vi "(SubVI)DW7914.vi"() -> ()   [LabVIEW 2020]
uses:
  Controls/(Ctrl)DW7914_Trig Wave Ctrl.ctl
  DW7912/Controls/(Ctrl)DW7912_Wave Seq.ctl
  System Command/Controls/(Ctrl)System Command_Trig GPIO Control.ctl
  <vilib>/Utility/miscctls.llb/LVPointTypeDef.ctl
  Control Data/Controls/(Ctrl)Control Data_Save or Load Control Data_Function.ctl
  Libraries/Haptic IC Class/Haptic IC/Haptic IC.lvclass/Haptic IC.ctl
  I2C/Controls/(Ctrl)I2C_8Bit_Read Array.ctl
  Waveform Editor/Controls/(Ctrl)Waveform Editor_Update Sampling Rate Value.ctl
  a7fdcbe2-e318-4fc3-ac41-e38a3fe8abb3.vi
  26a1efa9-de36-48db-9673-265351e4b95c.vi
  Libraries/Haptic IC Class/Haptic IC/Accessors/Write freq ref.vi
  Libraries/Haptic IC Class/Haptic IC/Accessors/Write voltage range ref.vi
  Libraries/Haptic IC Class/Haptic IC/Accessors/Write mode ref.vi
  Variables/(Var)System Variables.vi
  I2C/Instance VIs/(SubVI)I2C_8Bit-8Bit_Read_Single.vi
  I2C/Instance VIs/(SubVI)I2C_8Bit-8Bit_Read_Sequential.vi
  I2C/Instance VIs/(SubVI)I2C_8Bit-8Bit_Write_Single.vi
  I2C/Instance VIs/(SubVI)I2C_8Bit-8Bit_Read_Array.vi
  I2C/Instance VIs/(SubVI)I2C_8Bit-8Bit_Write_Sequential.vi
  <vilib>/Comparison/Equal/Equal Functor/Equal Functor.lvclass
  Libraries/Haptic IC Class/Haptic IC/Haptic IC.lvclass
panel:
  in  "Stop":bool
  in  "Read All":bool
  in  "Mode Tab":T1(tab)
  in  "Mem_Brake_VD":u8(ring) caption="Brake1 M VD" items=["1.0", "0.5", "0.25", "0.25"]
  in  "Mem_Brake_Cycle 1":u8(ring) caption="Brake1 M Cycle" items=["1", "2", "3", "4", "5", "6", "7", "8"]
  in  "Mem_Brake_Cycle 0":u8(ring) caption="Brake0 M Cycle" items=["1", "2", "3", "4"]
  in  "Mem_Brake_Wave 1":u8(ring) caption="Brake1 M Wave" items=["Empty", "1", "2", "3", "4", "5", "6", "7", "8", "9", "10", "11", "12", "13", "14", "15", "16", "17", "18", "19", "20", "21", "22", "23", "24", "25", "26", "27", "28", "29", "30", "31", "32", "33", "34", "35", "36", "37", "38", "39", "40", "41", "42", "43", "44", "45", "46", "47", "48", "49", "50", "51", "52", "53", "54", "55", "56", "57", "58", "59", "60", "61", "62", "63", "64", "65", "66", "67", "68", "69", "70", "71", "72", "73", "74", "75", "76", "77", "78", "79", "80", "81", "82", "83", "84", "85", "86", "87", "88", "89", "90", "91", "92", "93", "94", "95", "96", "97", "98", "99", "100", "101", "102", "103", "104", "105", "106", "107", "108", "109", "110", "111", "112", "113", "114", "115", "116", "117", "118", "119", "120", "121", "122", "123", "124", "125", "126", "127"]
  in  "Mem_Brake_Wave 0":u8(ring) caption="Brake0 M Wave" items=["Empty", "1", "2", "3", "4", "5", "6", "7", "8", "9", "10", "11", "12", "13", "14", "15", "16", "17", "18", "19", "20", "21", "22", "23", "24", "25", "26", "27", "28", "29", "30", "31", "32", "33", "34", "35", "36", "37", "38", "39", "40", "41", "42", "43", "44", "45", "46", "47", "48", "49", "50", "51", "52", "53", "54", "55", "56", "57", "58", "59", "60", "61", "62", "63", "64", "65", "66", "67", "68", "69", "70", "71", "72", "73", "74", "75", "76", "77", "78", "79", "80", "81", "82", "83", "84", "85", "86", "87", "88", "89", "90", "91", "92", "93", "94", "95", "96", "97", "98", "99", "100", "101", "102", "103", "104", "105", "106", "107", "108", "109", "110", "111", "112", "113", "114", "115", "116", "117", "118", "119", "120", "121", "122", "123", "124", "125", "126", "127"]
  in  "Mem Set_Wave Seq Loop":T2 {"Loop 7" items=["X1", "X2", "X3", "X4", "X5", "X6", "X7", "X8", "X9", "X10", "X11", "X12", "X13", "X14", "X15", "Infinite"]; "Loop 6" items=["X1", "X2", "X3", "X4", "X5", "X6", "X7", "X8", "X9", "X10", "X11", "X12", "X13", "X14", "X15", "Infinite"]; "Loop 5" items=["X1", "X2", "X3", "X4", "X5", "X6", "X7", "X8", "X9", "X10", "X11", "X12", "X13", "X14", "X15", "Infinite"]; "Loop 4" items=["X1", "X2", "X3", "X4", "X5", "X6", "X7", "X8", "X9", "X10", "X11", "X12", "X13", "X14", "X15", "Infinite"]; "Loop 3" items=["X1", "X2", "X3", "X4", "X5", "X6", "X7", "X8", "X9", "X10", "X11", "X12", "X13", "X14", "X15", "Infinite"]; "Loop 2" items=["X1", "X2", "X3", "X4", "X5", "X6", "X7", "X8", "X9", "X10", "X11", "X12", "X13", "X14", "X15", "Infinite"]; "Loop 1" items=["X1", "X2", "X3", "X4", "X5", "X6", "X7", "X8", "X9", "X10", "X11", "X12", "X13", "X14", "X15", "Infinite"]; "Loop 0" items=["X1", "X2", "X3", "X4", "X5", "X6", "X7", "X8", "X9", "X10", "X11", "X12", "X13", "X14", "X15", "Infinite"]}
  in  "Mem_Stop":bool
  in  "Mem_Start":bool
  in  "Mem_Wave Seq":T4 caption="WAVE SEQUENCE" {"Wave Seq. 7"."Seq/Delay" items=["Empty", "1", "2", "3", "4", "5", "6", "7", "8", "9", "10", "11", "12", "13", "14", "15", "16", "17", "18", "19", "20", "21", "22", "23", "24", "25", "26", "27", "28", "29", "30", "31", "32", "33", "34", "35", "36", "37", "38", "39", "40", "41", "42", "43", "44", "45", "46", "47", "48", "49", "50", "51", "52", "53", "54", "55", "56", "57", "58", "59", "60", "61", "62", "63", "64", "65", "66", "67", "68", "69", "70", "71", "72", "73", "74", "75", "76", "77", "78", "79", "80", "81", "82", "83", "84", "85", "86", "87", "88", "89", "90", "91", "92", "93", "94", "95", "96", "97", "98", "99", "100", "101", "102", "103", "104", "105", "106", "107", "108", "109", "110", "111", "112", "113", "114", "115", "116", "117", "118", "119", "120", "121", "122", "123", "124", "125", "126", "127"]; "Wave Seq. 7"."Mode" items=["Wave Seq. 7", "Delay"]; "Wave Seq. 6"."Seq/Delay" items=["Empty", "1", "2", "3", "4", "5", "6", "7", "8", "9", "10", "11", "12", "13", "14", "15", "16", "17", "18", "19", "20", "21", "22", "23", "24", "25", "26", "27", "28", "29", "30", "31", "32", "33", "34", "35", "36", "37", "38", "39", "40", "41", "42", "43", "44", "45", "46", "47", "48", "49", "50", "51", "52", "53", "54", "55", "56", "57", "58", "59", "60", "61", "62", "63", "64", "65", "66", "67", "68", "69", "70", "71", "72", "73", "74", "75", "76", "77", "78", "79", "80", "81", "82", "83", "84", "85", "86", "87", "88", "89", "90", "91", "92", "93", "94", "95", "96", "97", "98", "99", "100", "101", "102", "103", "104", "105", "106", "107", "108", "109", "110", "111", "112", "113", "114", "115", "116", "117", "118", "119", "120", "121", "122", "123", "124", "125", "126", "127"]; "Wave Seq. 6"."Mode" items=["Wave Seq. 6", "Delay"]; "Wave Seq. 5"."Seq/Delay" items=["Empty", "1", "2", "3", "4", "5", "6", "7", "8", "9", "10", "11", "12", "13", "14", "15", "16", "17", "18", "19", "20", "21", "22", "23", "24", "25", "26", "27", "28", "29", "30", "31", "32", "33", "34", "35", "36", "37", "38", "39", "40", "41", "42", "43", "44", "45", "46", "47", "48", "49", "50", "51", "52", "53", "54", "55", "56", "57", "58", "59", "60", "61", "62", "63", "64", "65", "66", "67", "68", "69", "70", "71", "72", "73", "74", "75", "76", "77", "78", "79", "80", "81", "82", "83", "84", "85", "86", "87", "88", "89", "90", "91", "92", "93", "94", "95", "96", "97", "98", "99", "100", "101", "102", "103", "104", "105", "106", "107", "108", "109", "110", "111", "112", "113", "114", "115", "116", "117", "118", "119", "120", "121", "122", "123", "124", "125", "126", "127"]; "Wave Seq. 5"."Mode" items=["Wave Seq. 5", "Delay"]; "Wave Seq. 4"."Seq/Delay" items=["Empty", "1", "2", "3", "4", "5", "6", "7", "8", "9", "10", "11", "12", "13", "14", "15", "16", "17", "18", "19", "20", "21", "22", "23", "24", "25", "26", "27", "28", "29", "30", "31", "32", "33", "34", "35", "36", "37", "38", "39", "40", "41", "42", "43", "44", "45", "46", "47", "48", "49", "50", "51", "52", "53", "54", "55", "56", "57", "58", "59", "60", "61", "62", "63", "64", "65", "66", "67", "68", "69", "70", "71", "72", "73", "74", "75", "76", "77", "78", "79", "80", "81", "82", "83", "84", "85", "86", "87", "88", "89", "90", "91", "92", "93", "94", "95", "96", "97", "98", "99", "100", "101", "102", "103", "104", "105", "106", "107", "108", "109", "110", "111", "112", "113", "114", "115", "116", "117", "118", "119", "120", "121", "122", "123", "124", "125", "126", "127"]; "Wave Seq. 4"."Mode" items=["Wave Seq. 4", "Delay"]; "Wave Seq. 3"."Seq/Delay" items=["Empty", "1", "2", "3", "4", "5", "6", "7", "8", "9", "10", "11", "12", "13", "14", "15", "16", "17", "18", "19", "20", "21", "22", "23", "24", "25", "26", "27", "28", "29", "30", "31", "32", "33", "34", "35", "36", "37", "38", "39", "40", "41", "42", "43", "44", "45", "46", "47", "48", "49", "50", "51", "52", "53", "54", "55", "56", "57", "58", "59", "60", "61", "62", "63", "64", "65", "66", "67", "68", "69", "70", "71", "72", "73", "74", "75", "76", "77", "78", "79", "80", "81", "82", "83", "84", "85", "86", "87", "88", "89", "90", "91", "92", "93", "94", "95", "96", "97", "98", "99", "100", "101", "102", "103", "104", "105", "106", "107", "108", "109", "110", "111", "112", "113", "114", "115", "116", "117", "118", "119", "120", "121", "122", "123", "124", "125", "126", "127"]; "Wave Seq. 3"."Mode" items=["Wave Seq. 3", "Delay"]; "Wave Seq. 2"."Seq/Delay" items=["Empty", "1", "2", "3", "4", "5", "6", "7", "8", "9", "10", "11", "12", "13", "14", "15", "16", "17", "18", "19", "20", "21", "22", "23", "24", "25", "26", "27", "28", "29", "30", "31", "32", "33", "34", "35", "36", "37", "38", "39", "40", "41", "42", "43", "44", "45", "46", "47", "48", "49", "50", "51", "52", "53", "54", "55", "56", "57", "58", "59", "60", "61", "62", "63", "64", "65", "66", "67", "68", "69", "70", "71", "72", "73", "74", "75", "76", "77", "78", "79", "80", "81", "82", "83", "84", "85", "86", "87", "88", "89", "90", "91", "92", "93", "94", "95", "96", "97", "98", "99", "100", "101", "102", "103", "104", "105", "106", "107", "108", "109", "110", "111", "112", "113", "114", "115", "116", "117", "118", "119", "120", "121", "122", "123", "124", "125", "126", "127"]; "Wave Seq. 2"."Mode" items=["Wave Seq. 2", "Delay"]; "Wave Seq. 1"."Seq/Delay" items=["Empty", "1", "2", "3", "4", "5", "6", "7", "8", "9", "10", "11", "12", "13", "14", "15", "16", "17", "18", "19", "20", "21", "22", "23", "24", "25", "26", "27", "28", "29", "30", "31", "32", "33", "34", "35", "36", "37", "38", "39", "40", "41", "42", "43", "44", "45", "46", "47", "48", "49", "50", "51", "52", "53", "54", "55", "56", "57", "58", "59", "60", "61", "62", "63", "64", "65", "66", "67", "68", "69", "70", "71", "72", "73", "74", "75", "76", "77", "78", "79", "80", "81", "82", "83", "84", "85", "86", "87", "88", "89", "90", "91", "92", "93", "94", "95", "96", "97", "98", "99", "100", "101", "102", "103", "104", "105", "106", "107", "108", "109", "110", "111", "112", "113", "114", "115", "116", "117", "118", "119", "120", "121", "122", "123", "124", "125", "126", "127"]; "Wave Seq. 1"."Mode" items=["Wave Seq. 1", "Delay"]; "Wave Seq. 0"."Seq/Delay" items=["Empty", "1", "2", "3", "4", "5", "6", "7", "8", "9", "10", "11", "12", "13", "14", "15", "16", "17", "18", "19", "20", "21", "22", "23", "24", "25", "26", "27", "28", "29", "30", "31", "32", "33", "34", "35", "36", "37", "38", "39", "40", "41", "42", "43", "44", "45", "46", "47", "48", "49", "50", "51", "52", "53", "54", "55", "56", "57", "58", "59", "60", "61", "62", "63", "64", "65", "66", "67", "68", "69", "70", "71", "72", "73", "74", "75", "76", "77", "78", "79", "80", "81", "82", "83", "84", "85", "86", "87", "88", "89", "90", "91", "92", "93", "94", "95", "96", "97", "98", "99", "100", "101", "102", "103", "104", "105", "106", "107", "108", "109", "110", "111", "112", "113", "114", "115", "116", "117", "118", "119", "120", "121", "122", "123", "124", "125", "126", "127"]; "Wave Seq. 0"."Mode" items=["Wave Seq. 0", "Delay"]}
  in  "Mem_Main Seq Loop":u8(ring) caption="Sequence Loop" items=["X1", "X2", "X3", "X4", "X5", "X6", "X7", "X8", "X9", "X10", "X11", "X12", "X13", "X14", "X15", "Infinite"]
  in  "Mem_Read":bool caption="Memory Mode"
  in  "Com_Bst_Mem Gain":u8(ring) caption="MEM Gain" items=["100%", "87.5%", "75%", "62.5%", "50%", "37.5%", "25%", "12.5%"]
  in  "Com_Bst_Mute":bool
  in  "AT_LRA_F0 In":u16(ring) caption="LRA F0 In" items=["0Hz", "1Hz", "2Hz", "3Hz", "4Hz", "5Hz", "6Hz", "7Hz", "8Hz", "9Hz", "10Hz", "11Hz", "12Hz", "13Hz", "14Hz", "15Hz", "16Hz", "17Hz", "18Hz", "19Hz", "20Hz", "21Hz", "22Hz", "23Hz", "24Hz", "25Hz", "26Hz", "27Hz", "28Hz", "29Hz", "30Hz", "31Hz", "32Hz", "33Hz", "34Hz", "35Hz", "36Hz", "37Hz", "38Hz", "39Hz", "40Hz", "41Hz", "42Hz", "43Hz", "44Hz", "45Hz", "46Hz", "47Hz", "48Hz", "49Hz", "50Hz", "51Hz", "52Hz", "53Hz", "54Hz", "55Hz", "56Hz", "57Hz", "58Hz", "59Hz", "60Hz", "61Hz", "62Hz", "63Hz", "64Hz", "65Hz", "66Hz", "67Hz", "68Hz", "69Hz", "70Hz", "71Hz", "72Hz", "73Hz", "74Hz", "75Hz", "76Hz", "77Hz", "78Hz", "79Hz", "80Hz", "81Hz", "82Hz", "83Hz", "84Hz", "85Hz", "86Hz", "87Hz", "88Hz", "89Hz", "90Hz", "91Hz", "92Hz", "93Hz", "94Hz", "95Hz", "96Hz", "97Hz", "98Hz", "99Hz", "100Hz", "101Hz", "102Hz", "103Hz", "104Hz", "105Hz", "106Hz", "107Hz", "108Hz", "109Hz", "110Hz", "111Hz", "112Hz", "113Hz", "114Hz", "115Hz", "116Hz", "117Hz", "118Hz", "119Hz", "120Hz", "121Hz", "122Hz", "123Hz", "124Hz", "125Hz", "126Hz", "127Hz", "128Hz", "129Hz", "130Hz", "131Hz", "132Hz", "133Hz", "134Hz", "135Hz", "136Hz", "137Hz", "138Hz", "139Hz", "140Hz", "141Hz", "142Hz", "143Hz", "144Hz", "145Hz", "146Hz", "147Hz", "148Hz", "149Hz", "150Hz", "151Hz", "152Hz", "153Hz", "154Hz", "155Hz", "156Hz", "157Hz", "158Hz", "159Hz", "160Hz", "161Hz", "162Hz", "163Hz", "164Hz", "165Hz", "166Hz", "167Hz", "168Hz", "169Hz", "170Hz", "171Hz", "172Hz", "173Hz", "174Hz", "175Hz", "176Hz", "177Hz", "178Hz", "179Hz", "180Hz", "181Hz", "182Hz", "183Hz", "184Hz", "185Hz", "186Hz", "187Hz", "188Hz", "189Hz", "190Hz", "191Hz", "192Hz", "193Hz", "194Hz", "195Hz", "196Hz", "197Hz", "198Hz", "199Hz", "200Hz", "201Hz", "202Hz", "203Hz", "204Hz", "205Hz", "206Hz", "207Hz", "208Hz", "209Hz", "210Hz", "211Hz", "212Hz", "213Hz", "214Hz", "215Hz", "216Hz", "217Hz", "218Hz", "219Hz", "220Hz", "221Hz", "222Hz", "223Hz", "224Hz", "225Hz", "226Hz", "227Hz", "228Hz", "229Hz", "230Hz", "231Hz", "232Hz", "233Hz", "234Hz", "235Hz", "236Hz", "237Hz", "238Hz", "239Hz", "240Hz", "241Hz", "242Hz", "243Hz", "244Hz", "245Hz", "246Hz", "247Hz", "248Hz", "249Hz", "250Hz", "251Hz", "252Hz", "253Hz", "254Hz", "255Hz", "256Hz", "257Hz", "258Hz", "259Hz", "260Hz", "261Hz", "262Hz", "263Hz", "264Hz", "265Hz", "266Hz", "267Hz", "268Hz", "269Hz", "270Hz", "271Hz", "272Hz", "273Hz", "274Hz", "275Hz", "276Hz", "277Hz", "278Hz", "279Hz", "280Hz", "281Hz", "282Hz", "283Hz", "284Hz", "285Hz", "286Hz", "287Hz", "288Hz", "289Hz", "290Hz", "291Hz", "292Hz", "293Hz", "294Hz", "295Hz", "296Hz", "297Hz", "298Hz", "299Hz", "300Hz", "301Hz", "302Hz", "303Hz", "304Hz", "305Hz", "306Hz", "307Hz", "308Hz", "309Hz", "310Hz", "311Hz", "312Hz", "313Hz", "314Hz", "315Hz", "316Hz", "317Hz", "318Hz", "319Hz", "320Hz", "321Hz", "322Hz", "323Hz", "324Hz", "325Hz", "326Hz", "327Hz", "328Hz", "329Hz", "330Hz", "331Hz", "332Hz", "333Hz", "334Hz", "335Hz", "336Hz", "337Hz", "338Hz", "339Hz", "340Hz", "341Hz", "342Hz", "343Hz", "344Hz", "345Hz", "346Hz", "347Hz", "348Hz", "349Hz", "350Hz", "351Hz", "352Hz", "353Hz", "354Hz", "355Hz", "356Hz", "357Hz", "358Hz", "359Hz", "360Hz", "361Hz", "362Hz", "363Hz", "364Hz", "365Hz", "366Hz", "367Hz", "368Hz", "369Hz", "370Hz", "371Hz", "372Hz", "373Hz", "374Hz", "375Hz", "376Hz", "377Hz", "378Hz", "379Hz", "380Hz", "381Hz", "382Hz", "383Hz", "384Hz", "385Hz", "386Hz", "387Hz", "388Hz", "389Hz", "390Hz", "391Hz", "392Hz", "393Hz", "394Hz", "395Hz", "396Hz", "397Hz", "398Hz", "399Hz", "400Hz", "401Hz", "402Hz", "403Hz", "404Hz", "405Hz", "406Hz", "407Hz", "408Hz", "409Hz", "410Hz", "411Hz", "412Hz", "413Hz", "414Hz", "415Hz", "416Hz", "417Hz", "418Hz", "419Hz", "420Hz", "421Hz", "422Hz", "423Hz", "424Hz", "425Hz", "426Hz", "427Hz", "428Hz", "429Hz", "430Hz", "431Hz", "432Hz", "433Hz", "434Hz", "435Hz", "436Hz", "437Hz", "438Hz", "439Hz", "440Hz", "441Hz", "442Hz", "443Hz", "444Hz", "445Hz", "446Hz", "447Hz", "448Hz", "449Hz", "450Hz", "451Hz", "452Hz", "453Hz", "454Hz", "455Hz", "456Hz", "457Hz", "458Hz", "459Hz", "460Hz", "461Hz", "462Hz", "463Hz", "464Hz", "465Hz", "466Hz", "467Hz", "468Hz", "469Hz", "470Hz", "471Hz", "472Hz", "473Hz", "474Hz", "475Hz", "476Hz", "477Hz", "478Hz", "479Hz", "480Hz", "481Hz", "482Hz", "483Hz", "484Hz", "485Hz", "486Hz", "487Hz", "488Hz", "489Hz", "490Hz", "491Hz", "492Hz", "493Hz", "494Hz", "495Hz", "496Hz", "497Hz", "498Hz", "499Hz", "500Hz", "501Hz", "502Hz", "503Hz", "504Hz", "505Hz", "506Hz", "507Hz", "508Hz", "509Hz", "510Hz", "511Hz"]
  in  "AT_LRA_F0":bool=TRUE
  in  "AT_Brake_VD":u8(ring) caption="Brake1 AT VD" items=["1.0", "0.5", "0.25", "0.25"]
  in  "AT_Brake_Cycle 1":u8(ring)=2 caption="Brake1 AT Cycle" items=["1", "2", "3", "4", "5", "6", "7", "8"]
  in  "AT_Brake_Cycle 0":u8(ring) caption="Brake0 AT Cycle" items=["1", "2", "3", "4"]
  in  "AT_Brake_Wave 1":u8(ring) caption="Brake1 AT Wave" items=["Empty", "1", "2", "3", "4", "5", "6", "7", "8", "9", "10", "11", "12", "13", "14", "15", "16", "17", "18", "19", "20", "21", "22", "23", "24", "25", "26", "27", "28", "29", "30", "31", "32", "33", "34", "35", "36", "37", "38", "39", "40", "41", "42", "43", "44", "45", "46", "47", "48", "49", "50", "51", "52", "53", "54", "55", "56", "57", "58", "59", "60", "61", "62", "63", "64", "65", "66", "67", "68", "69", "70", "71", "72", "73", "74", "75", "76", "77", "78", "79", "80", "81", "82", "83", "84", "85", "86", "87", "88", "89", "90", "91", "92", "93", "94", "95", "96", "97", "98", "99", "100", "101", "102", "103", "104", "105", "106", "107", "108", "109", "110", "111", "112", "113", "114", "115", "116", "117", "118", "119", "120", "121", "122", "123", "124", "125", "126", "127"]
  in  "AT_Brake_Wave 0":u8(ring) caption="Brake0 AT Wave" items=["Empty", "1", "2", "3", "4", "5", "6", "7", "8", "9", "10", "11", "12", "13", "14", "15", "16", "17", "18", "19", "20", "21", "22", "23", "24", "25", "26", "27", "28", "29", "30", "31", "32", "33", "34", "35", "36", "37", "38", "39", "40", "41", "42", "43", "44", "45", "46", "47", "48", "49", "50", "51", "52", "53", "54", "55", "56", "57", "58", "59", "60", "61", "62", "63", "64", "65", "66", "67", "68", "69", "70", "71", "72", "73", "74", "75", "76", "77", "78", "79", "80", "81", "82", "83", "84", "85", "86", "87", "88", "89", "90", "91", "92", "93", "94", "95", "96", "97", "98", "99", "100", "101", "102", "103", "104", "105", "106", "107", "108", "109", "110", "111", "112", "113", "114", "115", "116", "117", "118", "119", "120", "121", "122", "123", "124", "125", "126", "127"]
  in  "AT_Track_Wave 1":u8(ring) caption="Track1 Wave" items=["Empty", "1", "2", "3", "4", "5", "6", "7", "8", "9", "10", "11", "12", "13", "14", "15", "16", "17", "18", "19", "20", "21", "22", "23", "24", "25", "26", "27", "28", "29", "30", "31", "32", "33", "34", "35", "36", "37", "38", "39", "40", "41", "42", "43", "44", "45", "46", "47", "48", "49", "50", "51", "52", "53", "54", "55", "56", "57", "58", "59", "60", "61", "62", "63", "64", "65", "66", "67", "68", "69", "70", "71", "72", "73", "74", "75", "76", "77", "78", "79", "80", "81", "82", "83", "84", "85", "86", "87", "88", "89", "90", "91", "92", "93", "94", "95", "96", "97", "98", "99", "100", "101", "102", "103", "104", "105", "106", "107", "108", "109", "110", "111", "112", "113", "114", "115", "116", "117", "118", "119", "120", "121", "122", "123", "124", "125", "126", "127"]
  in  "AT_Track_Wave 0":u8(ring) caption="Track0 Wave" items=["Empty", "1", "2", "3", "4", "5", "6", "7", "8", "9", "10", "11", "12", "13", "14", "15", "16", "17", "18", "19", "20", "21", "22", "23", "24", "25", "26", "27", "28", "29", "30", "31", "32", "33", "34", "35", "36", "37", "38", "39", "40", "41", "42", "43", "44", "45", "46", "47", "48", "49", "50", "51", "52", "53", "54", "55", "56", "57", "58", "59", "60", "61", "62", "63", "64", "65", "66", "67", "68", "69", "70", "71", "72", "73", "74", "75", "76", "77", "78", "79", "80", "81", "82", "83", "84", "85", "86", "87", "88", "89", "90", "91", "92", "93", "94", "95", "96", "97", "98", "99", "100", "101", "102", "103", "104", "105", "106", "107", "108", "109", "110", "111", "112", "113", "114", "115", "116", "117", "118", "119", "120", "121", "122", "123", "124", "125", "126", "127"]
  in  "AT_Track_Idle":u8(ring) caption="Track Idle" items=["10.66ms", "21.32ms", "31.98ms", "42.64ms", "53.30ms", "63.96ms", "74.62ms", "85.28ms", "95.94ms", "106.60ms", "117.26ms", "127.92ms", "138.58ms", "149.24ms", "159.90ms", "170.56ms", "181.22ms", "191.88ms", "202.54ms", "213.20ms", "223.86ms", "234.52ms", "245.18ms", "255.84ms", "266.50ms", "277.16ms", "287.82ms", "298.48ms", "309.14ms", "319.80ms", "330.46ms", "341.12ms", "351.78ms", "362.44ms", "373.10ms", "383.76ms", "394.42ms", "405.08ms", "415.74ms", "426.40ms", "437.06ms", "447.72ms", "458.38ms", "469.04ms", "479.70ms", "490.36ms", "501.02ms", "511.68ms", "522.34ms", "533.00ms", "543.66ms", "554.32ms", "564.98ms", "575.64ms", "586.30ms", "596.96ms", "607.62ms", "618.28ms", "628.94ms", "639.60ms", "650.26ms", "660.92ms", "671.58ms", "682.24ms", "692.90ms", "703.56ms", "714.22ms", "724.88ms", "735.54ms", "746.20ms", "756.86ms", "767.52ms", "778.18ms", "788.84ms", "799.50ms", "810.16ms", "820.82ms", "831.48ms", "842.14ms", "852.80ms", "863.46ms", "874.12ms", "884.78ms", "895.44ms", "906.10ms", "916.76ms", "927.42ms", "938.08ms", "948.74ms", "959.40ms", "970.06ms", "980.72ms", "991.38ms", "1002.04ms", "1012.70ms", "1023.36ms", "1034.02ms", "1044.68ms", "1055.34ms", "1066.00ms", "1076.66ms", "1087.32ms", "1097.98ms", "1108.64ms", "1119.30ms", "1129.96ms", "1140.62ms", "1151.28ms", "1161.94ms", "1172.60ms", "1183.26ms", "1193.92ms", "1204.58ms", "1215.24ms", "1225.90ms", "1236.56ms", "1247.22ms", "1257.88ms", "1268.54ms", "1279.20ms", "1289.86ms", "1300.52ms", "1311.18ms", "1321.84ms", "1332.50ms", "1343.16ms", "1353.82ms", "1364.48ms", "1375.14ms", "1385.80ms", "1396.46ms", "1407.12ms", "1417.78ms", "1428.44ms", "1439.10ms", "1449.76ms", "1460.42ms", "1471.08ms", "1481.74ms", "1492.40ms", "1503.06ms", "1513.72ms", "1524.38ms", "1535.04ms", "1545.70ms", "1556.36ms", "1567.02ms", "1577.68ms", "1588.34ms", "1599.00ms", "1609.66ms", "1620.32ms", "1630.98ms", "1641.64ms", "1652.30ms", "1662.96ms", "1673.62ms", "1684.28ms", "1694.94ms", "1705.60ms", "1716.26ms", "1726.92ms", "1737.58ms", "1748.24ms", "1758.90ms", "1769.56ms", "1780.22ms", "1790.88ms", "1801.54ms", "1812.20ms", "1822.86ms", "1833.52ms", "1844.18ms", "1854.84ms", "1865.50ms", "1876.16ms", "1886.82ms", "1897.48ms", "1908.14ms", "1918.80ms", "1929.46ms", "1940.12ms", "1950.78ms", "1961.44ms", "1972.10ms", "1982.76ms", "1993.42ms", "2004.08ms", "2014.74ms", "2025.40ms", "2036.06ms", "2046.72ms", "2057.38ms", "2068.04ms", "2078.70ms", "2089.36ms", "2100.02ms", "2110.68ms", "2121.34ms", "2132.00ms", "2142.66ms", "2153.32ms", "2163.98ms", "2174.64ms", "2185.30ms", "2195.96ms", "2206.62ms", "2217.28ms", "2227.94ms", "2238.60ms", "2249.26ms", "2259.92ms", "2270.58ms", "2281.24ms", "2291.90ms", "2302.56ms", "2313.22ms", "2323.88ms", "2334.54ms", "2345.20ms", "2355.86ms", "2366.52ms", "2377.18ms", "2387.84ms", "2398.50ms", "2409.16ms", "2419.82ms", "2430.48ms", "2441.14ms", "2451.80ms", "2462.46ms", "2473.12ms", "2483.78ms", "2494.44ms", "2505.10ms", "2515.76ms", "2526.42ms", "2537.08ms", "2547.74ms", "2558.40ms", "2569.06ms", "2579.72ms", "2590.38ms", "2601.04ms", "2611.70ms", "2622.36ms", "2633.02ms", "2643.68ms", "2654.34ms", "2665.00ms", "2675.66ms", "2686.32ms", "2696.98ms", "2707.64ms", "2718.30ms", "2728.96ms"]
  in  "AT_Track_Play":u8(ring) caption="Track Play" items=["10.66ms", "21.32ms", "31.98ms", "42.64ms", "53.30ms", "63.96ms", "74.62ms", "85.28ms", "95.94ms", "106.60ms", "117.26ms", "127.92ms", "138.58ms", "149.24ms", "159.90ms", "170.56ms", "181.22ms", "191.88ms", "202.54ms", "213.20ms", "223.86ms", "234.52ms", "245.18ms", "255.84ms", "266.50ms", "277.16ms", "287.82ms", "298.48ms", "309.14ms", "319.80ms", "330.46ms", "341.12ms", "351.78ms", "362.44ms", "373.10ms", "383.76ms", "394.42ms", "405.08ms", "415.74ms", "426.40ms", "437.06ms", "447.72ms", "458.38ms", "469.04ms", "479.70ms", "490.36ms", "501.02ms", "511.68ms", "522.34ms", "533.00ms", "543.66ms", "554.32ms", "564.98ms", "575.64ms", "586.30ms", "596.96ms", "607.62ms", "618.28ms", "628.94ms", "639.60ms", "650.26ms", "660.92ms", "671.58ms", "682.24ms", "692.90ms", "703.56ms", "714.22ms", "724.88ms", "735.54ms", "746.20ms", "756.86ms", "767.52ms", "778.18ms", "788.84ms", "799.50ms", "810.16ms", "820.82ms", "831.48ms", "842.14ms", "852.80ms", "863.46ms", "874.12ms", "884.78ms", "895.44ms", "906.10ms", "916.76ms", "927.42ms", "938.08ms", "948.74ms", "959.40ms", "970.06ms", "980.72ms", "991.38ms", "1002.04ms", "1012.70ms", "1023.36ms", "1034.02ms", "1044.68ms", "1055.34ms", "1066.00ms", "1076.66ms", "1087.32ms", "1097.98ms", "1108.64ms", "1119.30ms", "1129.96ms", "1140.62ms", "1151.28ms", "1161.94ms", "1172.60ms", "1183.26ms", "1193.92ms", "1204.58ms", "1215.24ms", "1225.90ms", "1236.56ms", "1247.22ms", "1257.88ms", "1268.54ms", "1279.20ms", "1289.86ms", "1300.52ms", "1311.18ms", "1321.84ms", "1332.50ms", "1343.16ms", "1353.82ms", "1364.48ms", "1375.14ms", "1385.80ms", "1396.46ms", "1407.12ms", "1417.78ms", "1428.44ms", "1439.10ms", "1449.76ms", "1460.42ms", "1471.08ms", "1481.74ms", "1492.40ms", "1503.06ms", "1513.72ms", "1524.38ms", "1535.04ms", "1545.70ms", "1556.36ms", "1567.02ms", "1577.68ms", "1588.34ms", "1599.00ms", "1609.66ms", "1620.32ms", "1630.98ms", "1641.64ms", "1652.30ms", "1662.96ms", "1673.62ms", "1684.28ms", "1694.94ms", "1705.60ms", "1716.26ms", "1726.92ms", "1737.58ms", "1748.24ms", "1758.90ms", "1769.56ms", "1780.22ms", "1790.88ms", "1801.54ms", "1812.20ms", "1822.86ms", "1833.52ms", "1844.18ms", "1854.84ms", "1865.50ms", "1876.16ms", "1886.82ms", "1897.48ms", "1908.14ms", "1918.80ms", "1929.46ms", "1940.12ms", "1950.78ms", "1961.44ms", "1972.10ms", "1982.76ms", "1993.42ms", "2004.08ms", "2014.74ms", "2025.40ms", "2036.06ms", "2046.72ms", "2057.38ms", "2068.04ms", "2078.70ms", "2089.36ms", "2100.02ms", "2110.68ms", "2121.34ms", "2132.00ms", "2142.66ms", "2153.32ms", "2163.98ms", "2174.64ms", "2185.30ms", "2195.96ms", "2206.62ms", "2217.28ms", "2227.94ms", "2238.60ms", "2249.26ms", "2259.92ms", "2270.58ms", "2281.24ms", "2291.90ms", "2302.56ms", "2313.22ms", "2323.88ms", "2334.54ms", "2345.20ms", "2355.86ms", "2366.52ms", "2377.18ms", "2387.84ms", "2398.50ms", "2409.16ms", "2419.82ms", "2430.48ms", "2441.14ms", "2451.80ms", "2462.46ms", "2473.12ms", "2483.78ms", "2494.44ms", "2505.10ms", "2515.76ms", "2526.42ms", "2537.08ms", "2547.74ms", "2558.40ms", "2569.06ms", "2579.72ms", "2590.38ms", "2601.04ms", "2611.70ms", "2622.36ms", "2633.02ms", "2643.68ms", "2654.34ms", "2665.00ms", "2675.66ms", "2686.32ms", "2696.98ms", "2707.64ms", "2718.30ms", "Infinite"]
  in  "AT_Track_Cycle 0":u8(ring) caption="Track0 Cycle" items=["1", "2", "3", "4", "5", "6", "7", "8"]
  in  "AT_Track_Loop":u8(ring) caption="Track Loop" items=["X1", "X2", "X3", "X4", "X5", "X6", "X7", "X8", "X9", "X10", "X11", "X12", "X13", "X14", "X15", "Infinite"]
  in  "AT_Track_Pattern":bool=TRUE
  in  "AT_Read":bool caption="Auto Track Mode"
  in  "AT_Start":bool
  in  "AT_Stop":bool
  out "Trig_Gen_Pict":picture
  in  "Trig_Ctrl_Interval":u8(ring)=2 caption="TRIG Interval" items=["2.5ms", "5ms", "10ms", "20ms", "40ms", "60ms", "80ms", "100ms"]
  in  "Trig_Ctrl_Tirg1 Mode":bool
  in  "Trig_Ctrl_Sound Mode":bool
  in  "Trig_Ctrl_Trig2 Master":bool
  in  "Trig_Ctrl_Trig1 Level":bool
  in  "Trig_Ctrl_Trig Priority":bool
  in  "Trig_Gen_Set":bool
  in  "Trig_Gen_Setting":T5={"1st Trig"={"Trigger"=TRUE, "Low"=0, "High"=100}, "2nd Trig"={"Trigger"=TRUE, "Low"=0, "High"=100}, "3rd Trig"={"Trigger"=TRUE, "Low"=0, "High"=100}, "4th Trig"={"Trigger"=FALSE, "Low"=0, "High"=1}} {"4th Trig"."High" min=1 max=8000; "4th Trig"."Low" max=7999; "3rd Trig"."High" min=1 max=8000; "3rd Trig"."Low" max=7999; "2nd Trig"."High" min=1 max=8000; "2nd Trig"."Low" max=7999; "1st Trig"."High" min=1 max=7410; "1st Trig"."Low" max=7999}
  in  "Trig_Wave_Type Tab":enum32{"TRIG1", "TRIG2", "TRIG3"}(tab) caption="TRIG1/2/3 WAVE CTRL"
  in  "Trig_Wave_Trig 1":T6={"TRIG R WAV"=0, "BRAKE0 R WAVE"=0, "BRAKE1 R WAVE"=0, "TRIG F WAV"=0, "BRAKE0 F WAVE"=0, "BRAKE1 F WAVE"=0, "BRAKE1 AT VD"=0, "BRAKE1 AT CYCLE"=2, "BRAKE0 AT CYCLE"=0} {"TRIG F WAV" items=["Empty", "1", "2", "3", "4", "5", "6", "7", "8", "9", "10", "11", "12", "13", "14", "15", "16", "17", "18", "19", "20", "21", "22", "23", "24", "25", "26", "27", "28", "29", "30", "31", "32", "33", "34", "35", "36", "37", "38", "39", "40", "41", "42", "43", "44", "45", "46", "47", "48", "49", "50", "51", "52", "53", "54", "55", "56", "57", "58", "59", "60", "61", "62", "63", "64", "65", "66", "67", "68", "69", "70", "71", "72", "73", "74", "75", "76", "77", "78", "79", "80", "81", "82", "83", "84", "85", "86", "87", "88", "89", "90", "91", "92", "93", "94", "95", "96", "97", "98", "99", "100", "101", "102", "103", "104", "105", "106", "107", "108", "109", "110", "111", "112", "113", "114", "115", "116", "117", "118", "119", "120", "121", "122", "123", "124", "125", "126", "127"]; "TRIG R WAV" items=["Empty", "1", "2", "3", "4", "5", "6", "7", "8", "9", "10", "11", "12", "13", "14", "15", "16", "17", "18", "19", "20", "21", "22", "23", "24", "25", "26", "27", "28", "29", "30", "31", "32", "33", "34", "35", "36", "37", "38", "39", "40", "41", "42", "43", "44", "45", "46", "47", "48", "49", "50", "51", "52", "53", "54", "55", "56", "57", "58", "59", "60", "61", "62", "63", "64", "65", "66", "67", "68", "69", "70", "71", "72", "73", "74", "75", "76", "77", "78", "79", "80", "81", "82", "83", "84", "85", "86", "87", "88", "89", "90", "91", "92", "93", "94", "95", "96", "97", "98", "99", "100", "101", "102", "103", "104", "105", "106", "107", "108", "109", "110", "111", "112", "113", "114", "115", "116", "117", "118", "119", "120", "121", "122", "123", "124", "125", "126", "127"]; "BRAKE0 R WAVE" items=["Empty", "1", "2", "3", "4", "5", "6", "7", "8", "9", "10", "11", "12", "13", "14", "15", "16", "17", "18", "19", "20", "21", "22", "23", "24", "25", "26", "27", "28", "29", "30", "31", "32", "33", "34", "35", "36", "37", "38", "39", "40", "41", "42", "43", "44", "45", "46", "47", "48", "49", "50", "51", "52", "53", "54", "55", "56", "57", "58", "59", "60", "61", "62", "63", "64", "65", "66", "67", "68", "69", "70", "71", "72", "73", "74", "75", "76", "77", "78", "79", "80", "81", "82", "83", "84", "85", "86", "87", "88", "89", "90", "91", "92", "93", "94", "95", "96", "97", "98", "99", "100", "101", "102", "103", "104", "105", "106", "107", "108", "109", "110", "111", "112", "113", "114", "115", "116", "117", "118", "119", "120", "121", "122", "123", "124", "125", "126", "127"]; "BRAKE0 AT CYCLE" items=["1", "2", "3", "4"]; "BRAKE0 F WAVE" items=["Empty", "1", "2", "3", "4", "5", "6", "7", "8", "9", "10", "11", "12", "13", "14", "15", "16", "17", "18", "19", "20", "21", "22", "23", "24", "25", "26", "27", "28", "29", "30", "31", "32", "33", "34", "35", "36", "37", "38", "39", "40", "41", "42", "43", "44", "45", "46", "47", "48", "49", "50", "51", "52", "53", "54", "55", "56", "57", "58", "59", "60", "61", "62", "63", "64", "65", "66", "67", "68", "69", "70", "71", "72", "73", "74", "75", "76", "77", "78", "79", "80", "81", "82", "83", "84", "85", "86", "87", "88", "89", "90", "91", "92", "93", "94", "95", "96", "97", "98", "99", "100", "101", "102", "103", "104", "105", "106", "107", "108", "109", "110", "111", "112", "113", "114", "115", "116", "117", "118", "119", "120", "121", "122", "123", "124", "125", "126", "127"]; "BRAKE1 R WAVE" items=["Empty", "1", "2", "3", "4", "5", "6", "7", "8", "9", "10", "11", "12", "13", "14", "15", "16", "17", "18", "19", "20", "21", "22", "23", "24", "25", "26", "27", "28", "29", "30", "31", "32", "33", "34", "35", "36", "37", "38", "39", "40", "41", "42", "43", "44", "45", "46", "47", "48", "49", "50", "51", "52", "53", "54", "55", "56", "57", "58", "59", "60", "61", "62", "63", "64", "65", "66", "67", "68", "69", "70", "71", "72", "73", "74", "75", "76", "77", "78", "79", "80", "81", "82", "83", "84", "85", "86", "87", "88", "89", "90", "91", "92", "93", "94", "95", "96", "97", "98", "99", "100", "101", "102", "103", "104", "105", "106", "107", "108", "109", "110", "111", "112", "113", "114", "115", "116", "117", "118", "119", "120", "121", "122", "123", "124", "125", "126", "127"]; "BRAKE1 AT CYCLE" items=["1", "2", "3", "4", "5", "6", "7", "8"]; "BRAKE1 AT VD" items=["1.0", "0.5", "0.25", "0.25"]; "BRAKE1 F WAVE" items=["Empty", "1", "2", "3", "4", "5", "6", "7", "8", "9", "10", "11", "12", "13", "14", "15", "16", "17", "18", "19", "20", "21", "22", "23", "24", "25", "26", "27", "28", "29", "30", "31", "32", "33", "34", "35", "36", "37", "38", "39", "40", "41", "42", "43", "44", "45", "46", "47", "48", "49", "50", "51", "52", "53", "54", "55", "56", "57", "58", "59", "60", "61", "62", "63", "64", "65", "66", "67", "68", "69", "70", "71", "72", "73", "74", "75", "76", "77", "78", "79", "80", "81", "82", "83", "84", "85", "86", "87", "88", "89", "90", "91", "92", "93", "94", "95", "96", "97", "98", "99", "100", "101", "102", "103", "104", "105", "106", "107", "108", "109", "110", "111", "112", "113", "114", "115", "116", "117", "118", "119", "120", "121", "122", "123", "124", "125", "126", "127"]}
  in  "Trig_Wave_Trig 2":T6={"TRIG R WAV"=0, "BRAKE0 R WAVE"=0, "BRAKE1 R WAVE"=0, "TRIG F WAV"=0, "BRAKE0 F WAVE"=0, "BRAKE1 F WAVE"=0, "BRAKE1 AT VD"=0, "BRAKE1 AT CYCLE"=2, "BRAKE0 AT CYCLE"=0} {"TRIG F WAV" items=["Empty", "1", "2", "3", "4", "5", "6", "7", "8", "9", "10", "11", "12", "13", "14", "15", "16", "17", "18", "19", "20", "21", "22", "23", "24", "25", "26", "27", "28", "29", "30", "31", "32", "33", "34", "35", "36", "37", "38", "39", "40", "41", "42", "43", "44", "45", "46", "47", "48", "49", "50", "51", "52", "53", "54", "55", "56", "57", "58", "59", "60", "61", "62", "63", "64", "65", "66", "67", "68", "69", "70", "71", "72", "73", "74", "75", "76", "77", "78", "79", "80", "81", "82", "83", "84", "85", "86", "87", "88", "89", "90", "91", "92", "93", "94", "95", "96", "97", "98", "99", "100", "101", "102", "103", "104", "105", "106", "107", "108", "109", "110", "111", "112", "113", "114", "115", "116", "117", "118", "119", "120", "121", "122", "123", "124", "125", "126", "127"]; "TRIG R WAV" items=["Empty", "1", "2", "3", "4", "5", "6", "7", "8", "9", "10", "11", "12", "13", "14", "15", "16", "17", "18", "19", "20", "21", "22", "23", "24", "25", "26", "27", "28", "29", "30", "31", "32", "33", "34", "35", "36", "37", "38", "39", "40", "41", "42", "43", "44", "45", "46", "47", "48", "49", "50", "51", "52", "53", "54", "55", "56", "57", "58", "59", "60", "61", "62", "63", "64", "65", "66", "67", "68", "69", "70", "71", "72", "73", "74", "75", "76", "77", "78", "79", "80", "81", "82", "83", "84", "85", "86", "87", "88", "89", "90", "91", "92", "93", "94", "95", "96", "97", "98", "99", "100", "101", "102", "103", "104", "105", "106", "107", "108", "109", "110", "111", "112", "113", "114", "115", "116", "117", "118", "119", "120", "121", "122", "123", "124", "125", "126", "127"]; "BRAKE0 R WAVE" items=["Empty", "1", "2", "3", "4", "5", "6", "7", "8", "9", "10", "11", "12", "13", "14", "15", "16", "17", "18", "19", "20", "21", "22", "23", "24", "25", "26", "27", "28", "29", "30", "31", "32", "33", "34", "35", "36", "37", "38", "39", "40", "41", "42", "43", "44", "45", "46", "47", "48", "49", "50", "51", "52", "53", "54", "55", "56", "57", "58", "59", "60", "61", "62", "63", "64", "65", "66", "67", "68", "69", "70", "71", "72", "73", "74", "75", "76", "77", "78", "79", "80", "81", "82", "83", "84", "85", "86", "87", "88", "89", "90", "91", "92", "93", "94", "95", "96", "97", "98", "99", "100", "101", "102", "103", "104", "105", "106", "107", "108", "109", "110", "111", "112", "113", "114", "115", "116", "117", "118", "119", "120", "121", "122", "123", "124", "125", "126", "127"]; "BRAKE0 AT CYCLE" items=["1", "2", "3", "4"]; "BRAKE0 F WAVE" items=["Empty", "1", "2", "3", "4", "5", "6", "7", "8", "9", "10", "11", "12", "13", "14", "15", "16", "17", "18", "19", "20", "21", "22", "23", "24", "25", "26", "27", "28", "29", "30", "31", "32", "33", "34", "35", "36", "37", "38", "39", "40", "41", "42", "43", "44", "45", "46", "47", "48", "49", "50", "51", "52", "53", "54", "55", "56", "57", "58", "59", "60", "61", "62", "63", "64", "65", "66", "67", "68", "69", "70", "71", "72", "73", "74", "75", "76", "77", "78", "79", "80", "81", "82", "83", "84", "85", "86", "87", "88", "89", "90", "91", "92", "93", "94", "95", "96", "97", "98", "99", "100", "101", "102", "103", "104", "105", "106", "107", "108", "109", "110", "111", "112", "113", "114", "115", "116", "117", "118", "119", "120", "121", "122", "123", "124", "125", "126", "127"]; "BRAKE1 R WAVE" items=["Empty", "1", "2", "3", "4", "5", "6", "7", "8", "9", "10", "11", "12", "13", "14", "15", "16", "17", "18", "19", "20", "21", "22", "23", "24", "25", "26", "27", "28", "29", "30", "31", "32", "33", "34", "35", "36", "37", "38", "39", "40", "41", "42", "43", "44", "45", "46", "47", "48", "49", "50", "51", "52", "53", "54", "55", "56", "57", "58", "59", "60", "61", "62", "63", "64", "65", "66", "67", "68", "69", "70", "71", "72", "73", "74", "75", "76", "77", "78", "79", "80", "81", "82", "83", "84", "85", "86", "87", "88", "89", "90", "91", "92", "93", "94", "95", "96", "97", "98", "99", "100", "101", "102", "103", "104", "105", "106", "107", "108", "109", "110", "111", "112", "113", "114", "115", "116", "117", "118", "119", "120", "121", "122", "123", "124", "125", "126", "127"]; "BRAKE1 AT CYCLE" items=["1", "2", "3", "4", "5", "6", "7", "8"]; "BRAKE1 AT VD" items=["1.0", "0.5", "0.25", "0.25"]; "BRAKE1 F WAVE" items=["Empty", "1", "2", "3", "4", "5", "6", "7", "8", "9", "10", "11", "12", "13", "14", "15", "16", "17", "18", "19", "20", "21", "22", "23", "24", "25", "26", "27", "28", "29", "30", "31", "32", "33", "34", "35", "36", "37", "38", "39", "40", "41", "42", "43", "44", "45", "46", "47", "48", "49", "50", "51", "52", "53", "54", "55", "56", "57", "58", "59", "60", "61", "62", "63", "64", "65", "66", "67", "68", "69", "70", "71", "72", "73", "74", "75", "76", "77", "78", "79", "80", "81", "82", "83", "84", "85", "86", "87", "88", "89", "90", "91", "92", "93", "94", "95", "96", "97", "98", "99", "100", "101", "102", "103", "104", "105", "106", "107", "108", "109", "110", "111", "112", "113", "114", "115", "116", "117", "118", "119", "120", "121", "122", "123", "124", "125", "126", "127"]}
  in  "Trig_Wave_Trig 3":T6={"TRIG R WAV"=0, "BRAKE0 R WAVE"=0, "BRAKE1 R WAVE"=0, "TRIG F WAV"=0, "BRAKE0 F WAVE"=0, "BRAKE1 F WAVE"=0, "BRAKE1 AT VD"=0, "BRAKE1 AT CYCLE"=2, "BRAKE0 AT CYCLE"=0} {"TRIG F WAV" items=["Empty", "1", "2", "3", "4", "5", "6", "7", "8", "9", "10", "11", "12", "13", "14", "15", "16", "17", "18", "19", "20", "21", "22", "23", "24", "25", "26", "27", "28", "29", "30", "31", "32", "33", "34", "35", "36", "37", "38", "39", "40", "41", "42", "43", "44", "45", "46", "47", "48", "49", "50", "51", "52", "53", "54", "55", "56", "57", "58", "59", "60", "61", "62", "63", "64", "65", "66", "67", "68", "69", "70", "71", "72", "73", "74", "75", "76", "77", "78", "79", "80", "81", "82", "83", "84", "85", "86", "87", "88", "89", "90", "91", "92", "93", "94", "95", "96", "97", "98", "99", "100", "101", "102", "103", "104", "105", "106", "107", "108", "109", "110", "111", "112", "113", "114", "115", "116", "117", "118", "119", "120", "121", "122", "123", "124", "125", "126", "127"]; "TRIG R WAV" items=["Empty", "1", "2", "3", "4", "5", "6", "7", "8", "9", "10", "11", "12", "13", "14", "15", "16", "17", "18", "19", "20", "21", "22", "23", "24", "25", "26", "27", "28", "29", "30", "31", "32", "33", "34", "35", "36", "37", "38", "39", "40", "41", "42", "43", "44", "45", "46", "47", "48", "49", "50", "51", "52", "53", "54", "55", "56", "57", "58", "59", "60", "61", "62", "63", "64", "65", "66", "67", "68", "69", "70", "71", "72", "73", "74", "75", "76", "77", "78", "79", "80", "81", "82", "83", "84", "85", "86", "87", "88", "89", "90", "91", "92", "93", "94", "95", "96", "97", "98", "99", "100", "101", "102", "103", "104", "105", "106", "107", "108", "109", "110", "111", "112", "113", "114", "115", "116", "117", "118", "119", "120", "121", "122", "123", "124", "125", "126", "127"]; "BRAKE0 R WAVE" items=["Empty", "1", "2", "3", "4", "5", "6", "7", "8", "9", "10", "11", "12", "13", "14", "15", "16", "17", "18", "19", "20", "21", "22", "23", "24", "25", "26", "27", "28", "29", "30", "31", "32", "33", "34", "35", "36", "37", "38", "39", "40", "41", "42", "43", "44", "45", "46", "47", "48", "49", "50", "51", "52", "53", "54", "55", "56", "57", "58", "59", "60", "61", "62", "63", "64", "65", "66", "67", "68", "69", "70", "71", "72", "73", "74", "75", "76", "77", "78", "79", "80", "81", "82", "83", "84", "85", "86", "87", "88", "89", "90", "91", "92", "93", "94", "95", "96", "97", "98", "99", "100", "101", "102", "103", "104", "105", "106", "107", "108", "109", "110", "111", "112", "113", "114", "115", "116", "117", "118", "119", "120", "121", "122", "123", "124", "125", "126", "127"]; "BRAKE0 AT CYCLE" items=["1", "2", "3", "4"]; "BRAKE0 F WAVE" items=["Empty", "1", "2", "3", "4", "5", "6", "7", "8", "9", "10", "11", "12", "13", "14", "15", "16", "17", "18", "19", "20", "21", "22", "23", "24", "25", "26", "27", "28", "29", "30", "31", "32", "33", "34", "35", "36", "37", "38", "39", "40", "41", "42", "43", "44", "45", "46", "47", "48", "49", "50", "51", "52", "53", "54", "55", "56", "57", "58", "59", "60", "61", "62", "63", "64", "65", "66", "67", "68", "69", "70", "71", "72", "73", "74", "75", "76", "77", "78", "79", "80", "81", "82", "83", "84", "85", "86", "87", "88", "89", "90", "91", "92", "93", "94", "95", "96", "97", "98", "99", "100", "101", "102", "103", "104", "105", "106", "107", "108", "109", "110", "111", "112", "113", "114", "115", "116", "117", "118", "119", "120", "121", "122", "123", "124", "125", "126", "127"]; "BRAKE1 R WAVE" items=["Empty", "1", "2", "3", "4", "5", "6", "7", "8", "9", "10", "11", "12", "13", "14", "15", "16", "17", "18", "19", "20", "21", "22", "23", "24", "25", "26", "27", "28", "29", "30", "31", "32", "33", "34", "35", "36", "37", "38", "39", "40", "41", "42", "43", "44", "45", "46", "47", "48", "49", "50", "51", "52", "53", "54", "55", "56", "57", "58", "59", "60", "61", "62", "63", "64", "65", "66", "67", "68", "69", "70", "71", "72", "73", "74", "75", "76", "77", "78", "79", "80", "81", "82", "83", "84", "85", "86", "87", "88", "89", "90", "91", "92", "93", "94", "95", "96", "97", "98", "99", "100", "101", "102", "103", "104", "105", "106", "107", "108", "109", "110", "111", "112", "113", "114", "115", "116", "117", "118", "119", "120", "121", "122", "123", "124", "125", "126", "127"]; "BRAKE1 AT CYCLE" items=["1", "2", "3", "4", "5", "6", "7", "8"]; "BRAKE1 AT VD" items=["1.0", "0.5", "0.25", "0.25"]; "BRAKE1 F WAVE" items=["Empty", "1", "2", "3", "4", "5", "6", "7", "8", "9", "10", "11", "12", "13", "14", "15", "16", "17", "18", "19", "20", "21", "22", "23", "24", "25", "26", "27", "28", "29", "30", "31", "32", "33", "34", "35", "36", "37", "38", "39", "40", "41", "42", "43", "44", "45", "46", "47", "48", "49", "50", "51", "52", "53", "54", "55", "56", "57", "58", "59", "60", "61", "62", "63", "64", "65", "66", "67", "68", "69", "70", "71", "72", "73", "74", "75", "76", "77", "78", "79", "80", "81", "82", "83", "84", "85", "86", "87", "88", "89", "90", "91", "92", "93", "94", "95", "96", "97", "98", "99", "100", "101", "102", "103", "104", "105", "106", "107", "108", "109", "110", "111", "112", "113", "114", "115", "116", "117", "118", "119", "120", "121", "122", "123", "124", "125", "126", "127"]}
  in  "Trig_Read":bool caption="Trig Mode"
  in  "Common Tab":enum32{"Common"}(tab)
  in  "Com_Bst_Limit":u8(ring) caption="BST Limit" items=["3.0A", "3.5A", "4.0A", "2.5A"]
  out "Com_Status_Result":string caption="Result"
  in  "Com_Bst_VD Clamp":u8(ring) caption="VD Clamp" items=["0.00V", "0.04V", "0.08V", "0.12V", "0.16V", "0.20V", "0.24V", "0.28V", "0.32V", "0.36V", "0.40V", "0.44V", "0.48V", "0.52V", "0.56V", "0.60V", "0.64V", "0.68V", "0.72V", "0.76V", "0.80V", "0.84V", "0.88V", "0.92V", "0.96V", "1.00V", "1.04V", "1.08V", "1.12V", "1.16V", "1.20V", "1.24V", "1.28V", "1.32V", "1.36V", "1.40V", "1.44V", "1.48V", "1.52V", "1.56V", "1.60V", "1.64V", "1.68V", "1.72V", "1.76V", "1.80V", "1.84V", "1.88V", "1.92V", "1.96V", "2.00V", "2.04V", "2.08V", "2.12V", "2.16V", "2.20V", "2.24V", "2.28V", "2.32V", "2.36V", "2.40V", "2.44V", "2.48V", "2.52V", "2.56V", "2.60V", "2.64V", "2.68V", "2.72V", "2.76V", "2.80V", "2.84V", "2.88V", "2.92V", "2.96V", "3.00V", "3.04V", "3.08V", "3.12V", "3.16V", "3.20V", "3.24V", "3.28V", "3.32V", "3.36V", "3.40V", "3.44V", "3.48V", "3.52V", "3.56V", "3.60V", "3.64V", "3.68V", "3.72V", "3.76V", "3.80V", "3.84V", "3.88V", "3.92V", "3.96V", "4.00V", "4.04V", "4.08V", "4.12V", "4.16V", "4.20V", "4.24V", "4.28V", "4.32V", "4.36V", "4.40V", "4.44V", "4.48V", "4.52V", "4.56V", "4.60V", "4.64V", "4.68V", "4.72V", "4.76V", "4.80V", "4.84V", "4.88V", "4.92V", "4.96V", "5.00V", "5.04V", "5.08V", "5.12V", "5.16V", "5.20V", "5.24V", "5.28V", "5.32V", "5.36V", "5.40V", "5.44V", "5.48V", "5.52V", "5.56V", "5.60V", "5.64V", "5.68V", "5.72V", "5.76V", "5.80V", "5.84V", "5.88V", "5.92V", "5.96V", "6.00V", "6.04V", "6.08V", "6.12V", "6.16V", "6.20V", "6.24V", "6.28V", "6.32V", "6.36V", "6.40V", "6.44V", "6.48V", "6.52V", "6.56V", "6.60V", "6.64V", "6.68V", "6.72V", "6.76V", "6.80V", "6.84V", "6.88V", "6.92V", "6.96V", "7.00V", "7.04V", "7.08V", "7.12V", "7.16V", "7.20V", "7.24V", "7.28V", "7.32V", "7.36V", "7.40V", "7.44V", "7.48V", "7.52V", "7.56V", "7.60V", "7.64V", "7.68V", "7.72V", "7.76V", "7.80V", "7.84V", "7.88V", "7.92V", "7.96V", "8.00V", "8.04V", "8.08V", "8.12V", "8.16V", "8.20V", "8.24V", "8.28V", "8.32V", "8.36V", "8.40V", "8.44V", "8.48V", "8.52V", "8.56V", "8.60V", "8.64V", "8.68V", "8.72V", "8.76V", "8.80V", "8.84V", "8.88V", "8.92V", "8.96V", "9.00V", "9.04V", "9.08V", "9.12V", "9.16V", "9.20V", "9.24V", "9.28V", "9.32V", "9.36V", "9.40V", "9.44V", "9.48V", "9.52V", "9.56V", "9.60V", "9.64V", "9.68V", "9.72V", "9.76V", "9.80V", "9.84V", "9.88V", "9.92V", "9.96V", "10.00V", "10.04V", "10.08V", "10.12V", "10.16V", "10.20V"]
  in  "Com_Bst_Mode":u8(ring)=4 caption="Mode" items=["Bypass"=2, "Lump"=4, "Adapt"=8]
  in  "Com_Bst_Offset":u8(ring) caption="BST Offset" items=["0.00V", "0.08V", "0.16V", "0.24V", "0.32V", "0.40V", "0.48V", "0.56V", "0.64V", "0.72V", "0.80V", "0.88V", "0.96V", "1.04V", "1.12V", "1.20V"]
  in  "Com_Mode":T7 caption="MODE"
  in  "Com_Bst_Wait":u8(ring) caption="Wait Time" items=["0us", "166us", "332us", "498us", "664us", "830us", "996us", "1162us", "1328us", "1494us", "1660us", "1826us", "1992us", "2158us", "2324us", "2490us"]
  in  "Com_PWM_Mode":u8(ring) caption="VD Clamp Reg" items=["Header", "VD Clamp"]
  in  "Com_PWM_VHM":u8(ring) caption="VMH CTRL" items=["0", "1", "2", "3"]
  in  "Com_PWM_Freq":u8(ring)=1 caption="PWM Freq." items=["24kHz", "48kHz", "96kHz", "12kHz"]
  in  "Com_PWM_VD Time":u8(ring) caption="VD Clamp Time" items=["No Limit", "20ms", "40ms", "80ms"]
  in  "Com_Status_Select":T8(ring) caption="Select"
  in  "Com_Read":bool caption="Common"
  # "WAVE SEQ CTRL"
  # "MEM BRAKE CTRL"
  # "Wave Seq."
  # "Mem No."
  # "Loop"
  # "TRACK CTRL"
  # "BRAKE AT CTRL"
  # "LRA CTRL"
  # "TRIG CTRL"
  # "TRIGGER GENERATOR"
  # "Trigger"
  # "R (ms)"
  # "F (ms)"
  # "STATUS READ"
  # "PWM FREQ / ETC"
  # "BOOST MODE"
  # "VD CLAMP"
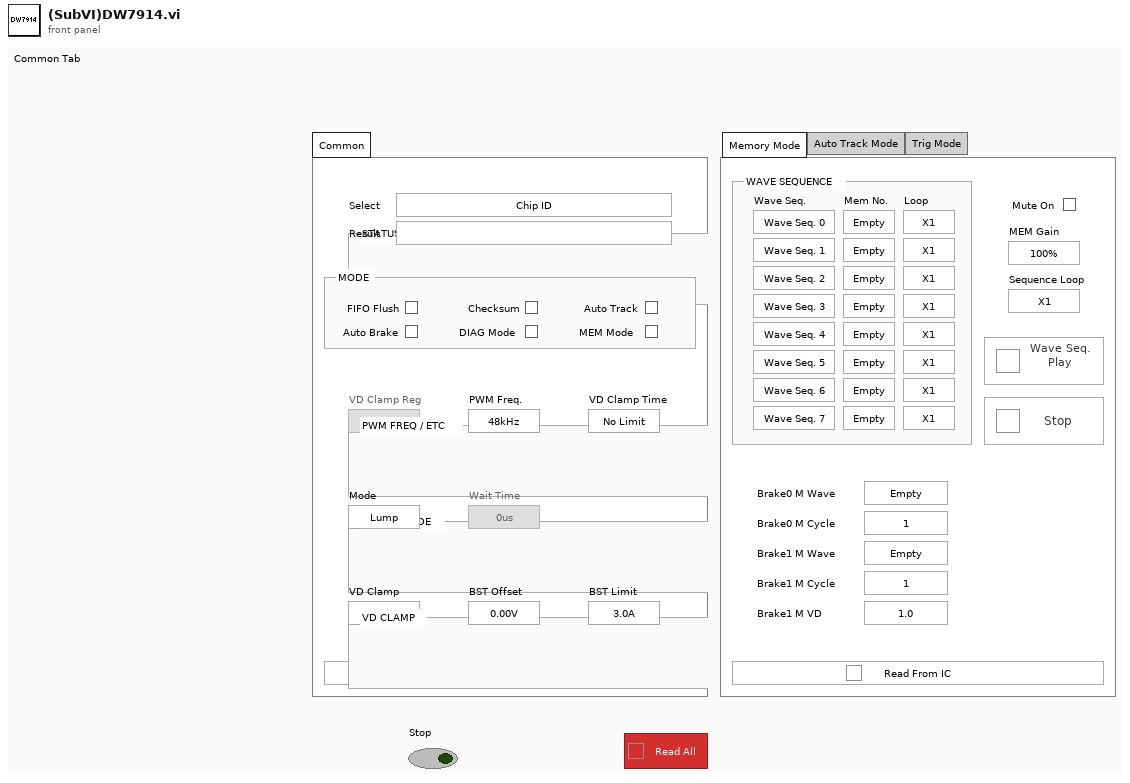
[diagram p1: front panel]
types:
  T1 = enum32{"Memory Mode", "Auto Track Mode", "Trig Mode"}
  T2 = cluster{"Loop 0":u8, "Loop 1":u8, "Loop 2":u8, "Loop 3":u8, "Loop 4":u8, "Loop 5":u8, "Loop 6":u8, "Loop 7":u8}
  T3 = typedef "(Ctrl)DW7912_Wave Seq.ctl" = cluster{"Mode":u8, "Seq/Delay":u8}
  T4 = cluster{"Wave Seq. 0":T3, "Wave Seq. 1":T3, "Wave Seq. 2":T3, "Wave Seq. 3":T3, "Wave Seq. 4":T3, "Wave Seq. 5":T3, "Wave Seq. 6":T3, "Wave Seq. 7":T3}
  T5 = typedef "(Ctrl)System Command_Trig GPIO Control.ctl" = cluster{"1st Trig":cluster{"Trigger":bool, "Low":u16, "High":u16}, "2nd Trig":cluster{"Trigger":bool, "Low":u16, "High":u16}, "3rd Trig":cluster{"Trigger":bool, "Low":u16, "High":u16}, "4th Trig":cluster{"Trigger":bool, "Low":u16, "High":u16}}
  T6 = typedef "(Ctrl)DW7914_Trig Wave Ctrl.ctl" = cluster{"TRIG R WAV":u8, "BRAKE0 R WAVE":u8, "BRAKE1 R WAVE":u8, "TRIG F WAV":u8, "BRAKE0 F WAVE":u8, "BRAKE1 F WAVE":u8, "BRAKE1 AT VD":u8, "BRAKE1 AT CYCLE":u8, "BRAKE0 AT CYCLE":u8}
  T7 = cluster{"MEM_MODE":bool, "DIAG_MODE":bool, "AUTO_BRAKE":bool, "AUTO_TRACK":bool, "CHKSUM":bool, "FIFO_FLUSH":bool}
  T8 = enum16{"Chip ID", "VBAT", "Status 0", "Status 1", "LRA F0 Value", "FIFO Status", "RAM Checksum", "FIFO Level", ""}
  T9 = enum8{"Enabled", "Disabled", "Disabled and Grayed Out"}
  T10 = typedef "(Ctrl)Control Data_Save or Load Control Data_Function.ctl" = enum16{"Save", "Load"}
  T11 = typedef "LVPointTypeDef.ctl" = cluster{"Horizontal":i16, "Vertical":i16}
  T12 = enum16{"CHIP ID", "VBAT", "STATUS 0", "STATUS 1", "LRA F0 VALUE", "FIFO STATUS", "RAM CHECKSUM", "FIFO LEVEL"}
  T13 = typedef "(Ctrl)I2C_8Bit_Read Array.ctl" = cluster{"Address":u8, "Delay(ms)":i32}
  T14 = typedef "(Ctrl)Waveform Editor_Update Sampling Rate Value.ctl" = enum16{"Init", "Update"}
  T15 = cluster{"Boolean array[0]":bool, "Boolean array[1]":bool, "Boolean array[2]":bool, "Boolean array[3]":bool, "Boolean array[4]":bool, "Boolean array[5]":bool}
  T16 = cluster{"[0]":cluster{u8, u8}, "[1]":cluster{u8, u8}, "[2]":cluster{u8, u8}, "[3]":cluster{u8, u8}, "[4]":cluster{u8, u8}, "[5]":cluster{u8, u8}, "[6]":cluster{u8, u8}, "[7]":cluster{u8, u8}}
  T17 = cluster{"[0]":u8, "[1]":u8, "[2]":u8, "[3]":u8, "[4]":u8, "[5]":u8, "[6]":u8, "[7]":u8}
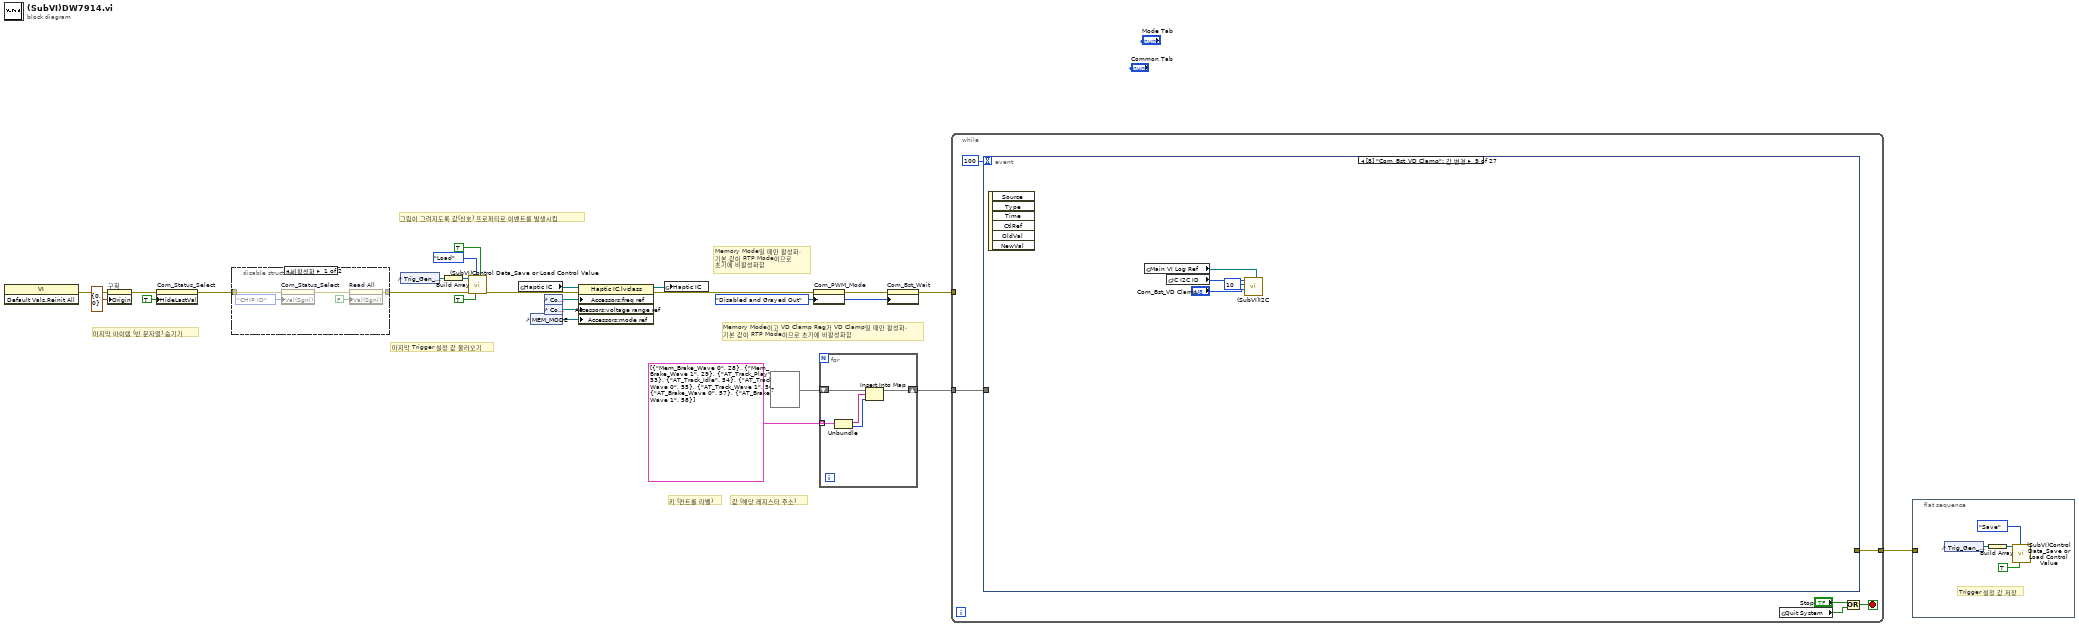
[diagram p0: block diagram]
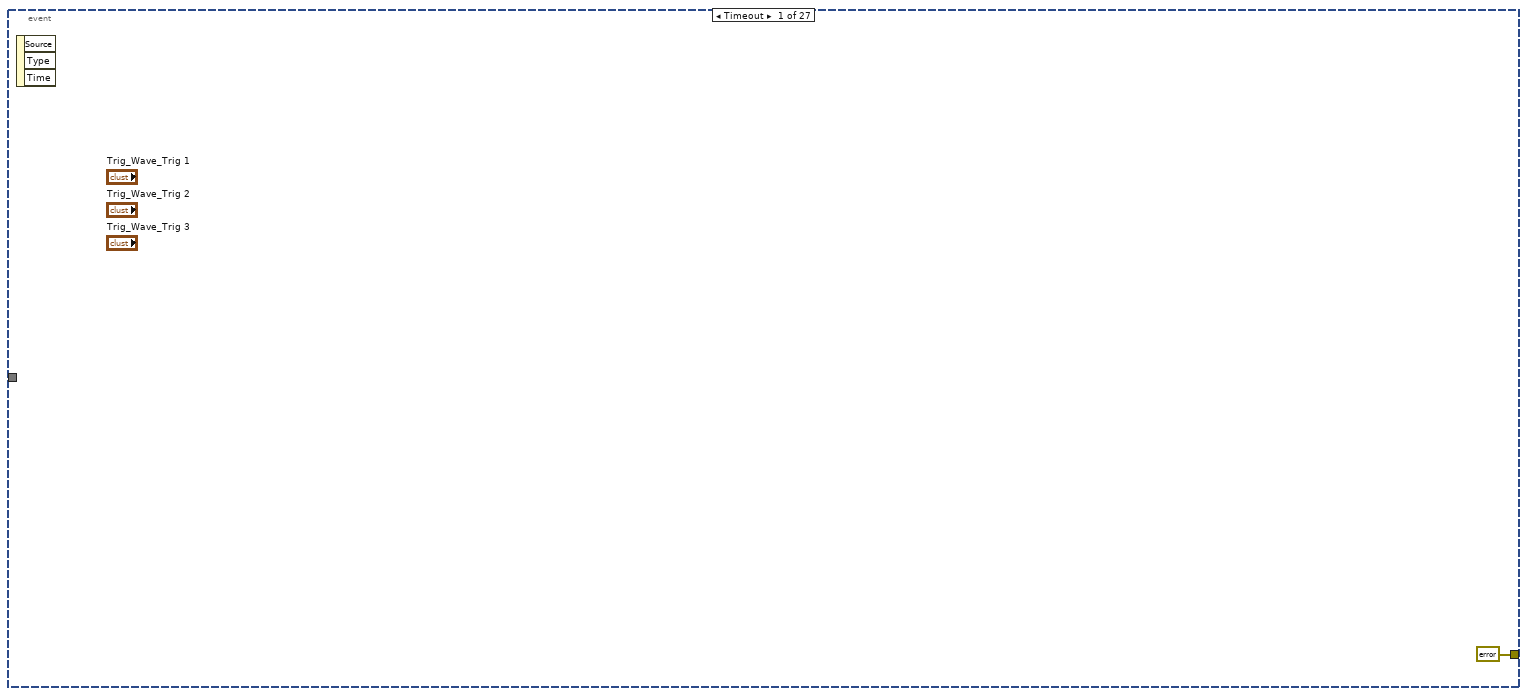
[diagram p3: hidden frame]
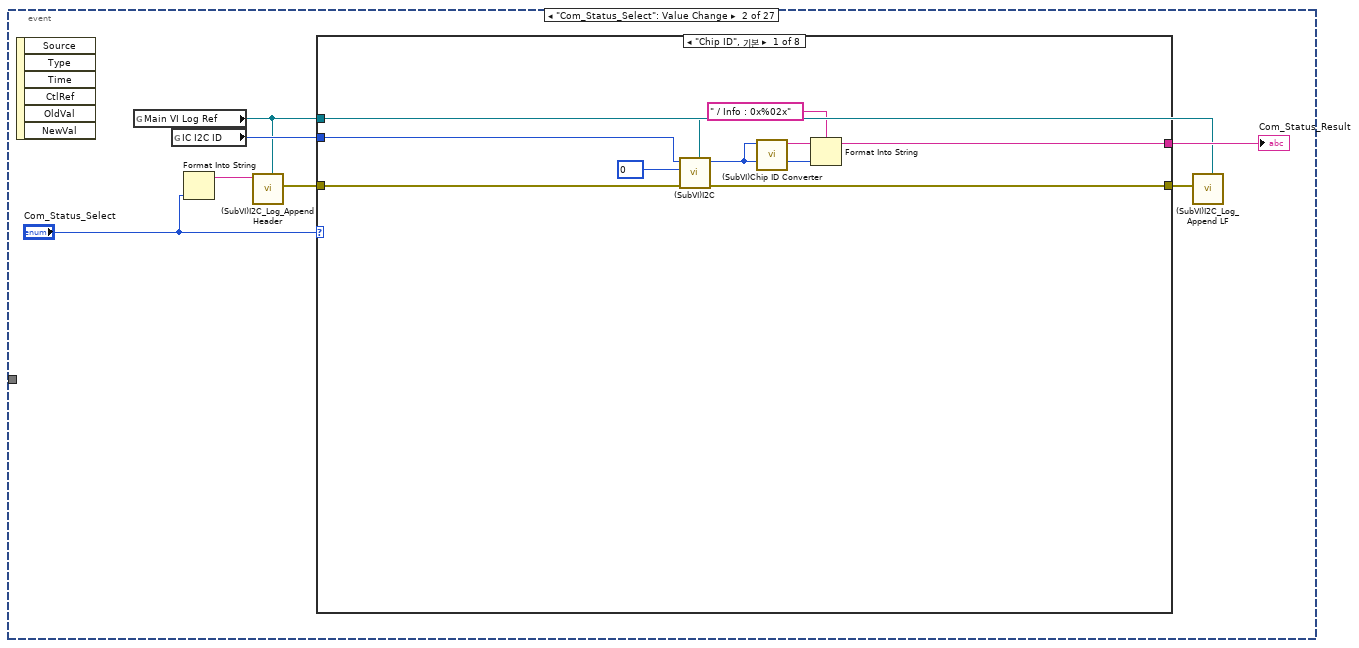
[diagram p4: hidden frame]
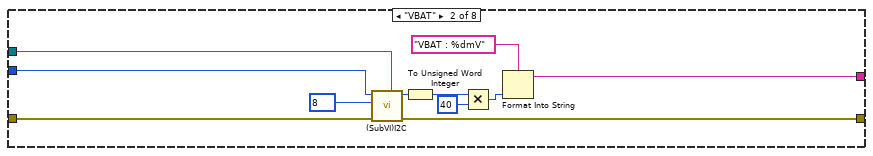
[diagram p5: hidden frame]
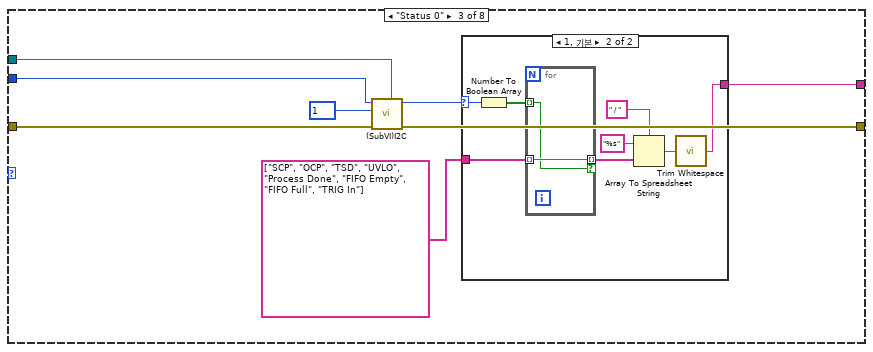
[diagram p6: hidden frame]
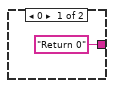
[diagram p7: hidden frame]
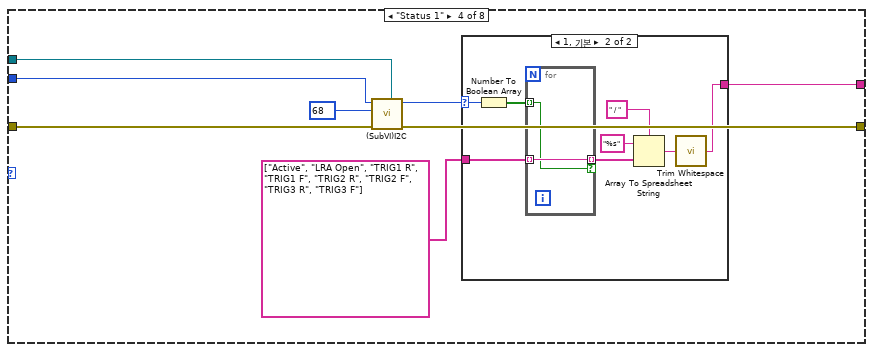
[diagram p8: hidden frame]
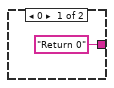
[diagram p9: hidden frame]
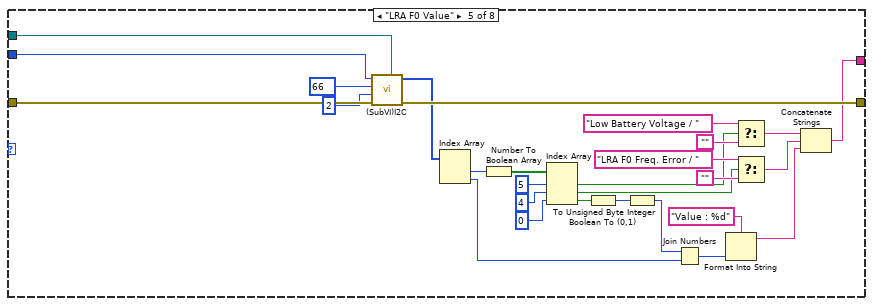
[diagram p10: hidden frame]
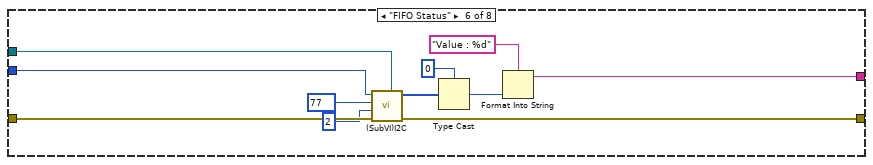
[diagram p11: hidden frame]
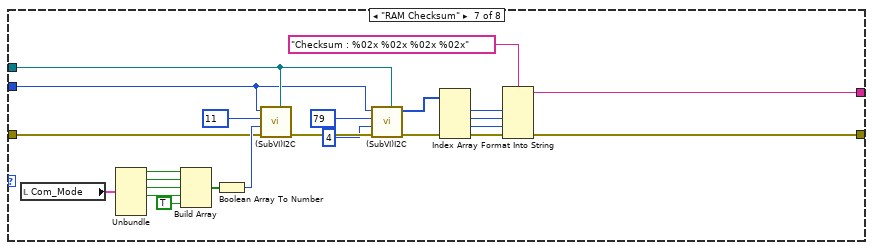
[diagram p12: hidden frame]
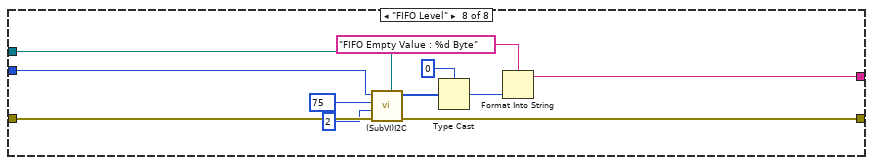
[diagram p13: hidden frame]
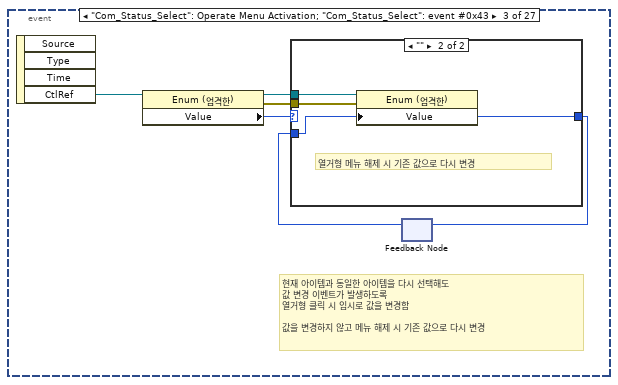
[diagram p14: hidden frame]
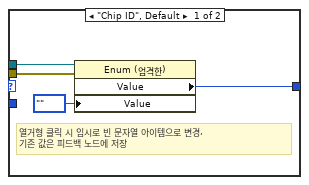
[diagram p15: hidden frame]
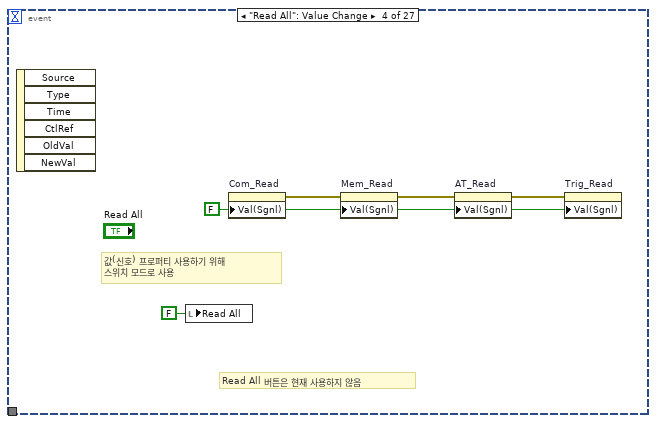
[diagram p16: hidden frame]
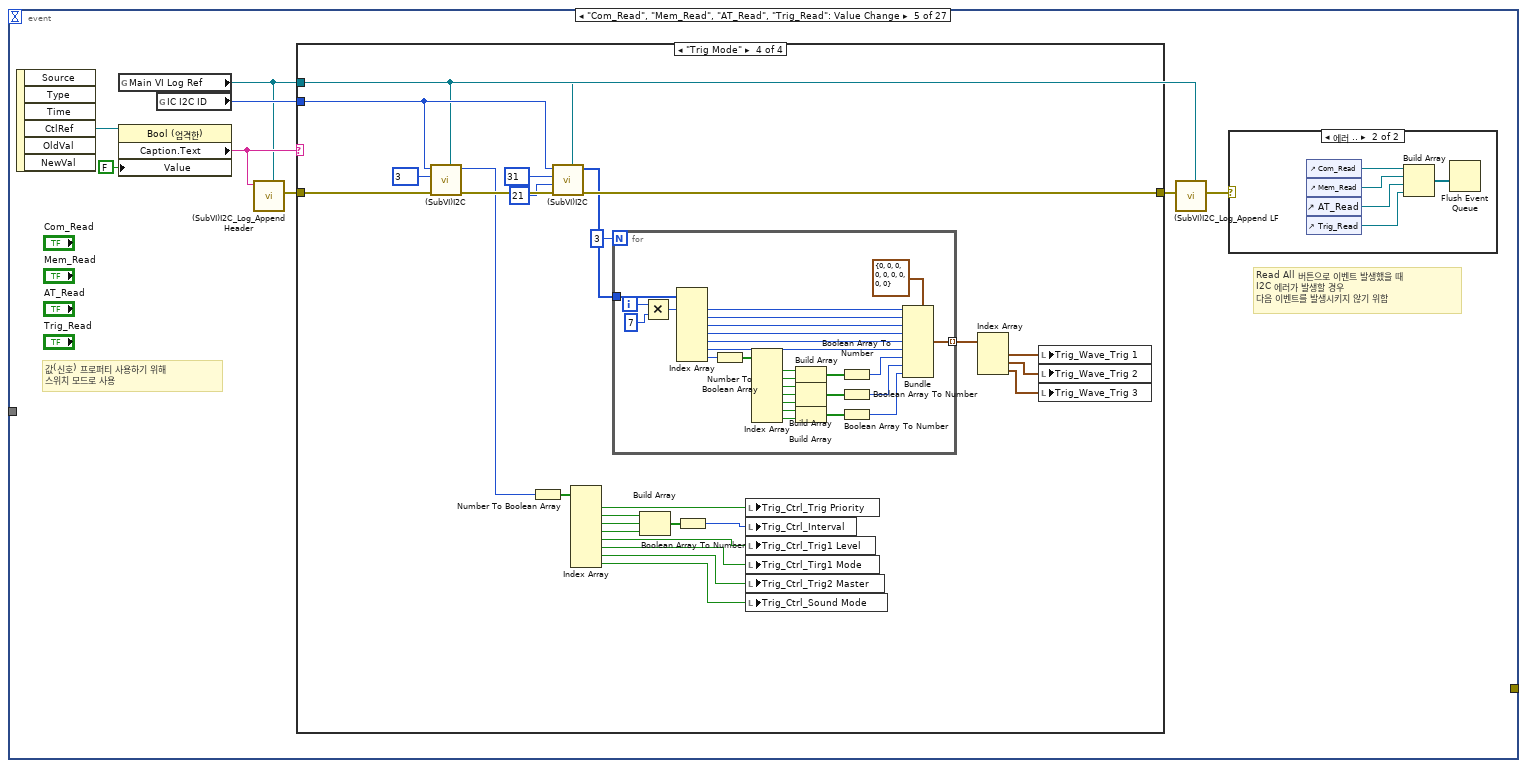
[diagram p17: hidden frame]
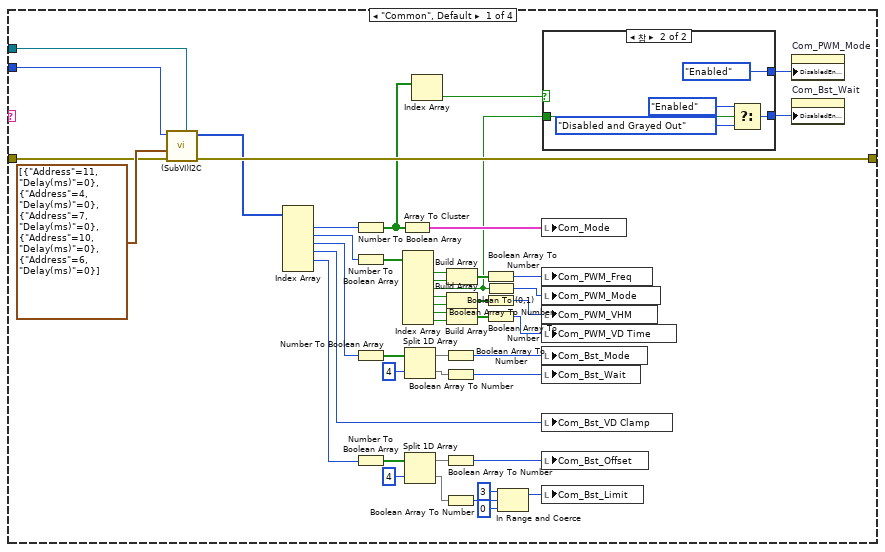
[diagram p18: hidden frame]
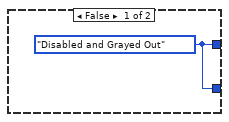
[diagram p19: hidden frame]
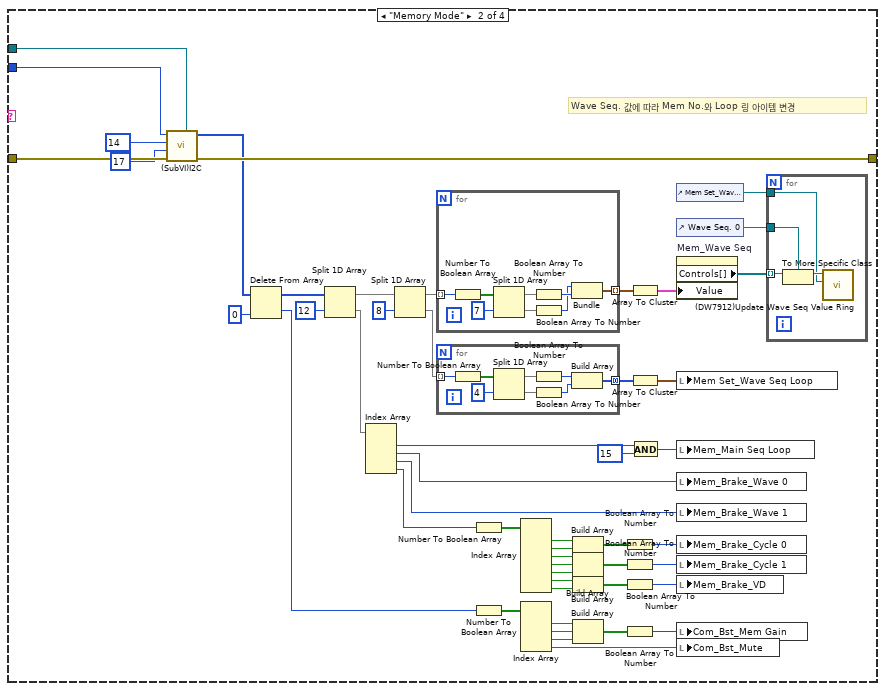
[diagram p20: hidden frame]
diagram:
  w2 = T9."Disabled and Grayed Out" ("비활성화")
  # "값 (해당 레지스터 주소)"
  # "키 (컨트롤 라벨)"
  # "Memory Mode이고 VD Clamp Reg가 VD Clamp일 때만 활성화,\n기본 값이 RTP Mode이므로 초기에 비활성화함"
  # "Memory Mode일 때만 활성화,\n기본 값이 RTP Mode이므로\n초기에 비활성화함"
  # "마지막 아이템 (빈 문자열) 숨기기"
  # "그림이 그려지도록 값(신호) 프로퍼티로 이벤트를 발생시킴"
  # "마지막 Trigger 설정 값 불러오기"
  n1 = invoke class="VI" method="Default Vals.Reinit All"() -> (error out=w25:errorcluster)  [unwired: 3 in, 2 out]
  n2 = property on="구획" class="Pane"(error in=w25, "Origin"=T11 {"Horizontal"=0, "Vertical"=0} ("원점")) -> (error out=w14:errorcluster)  [unwired: 1 in, 1 out]
  n3 = property on="Com_Status_Select" class="Enum (엄격한)"(error in=w14, "HideLastVal"=TRUE ("Hide Last Value")) -> (error out=w13:errorcluster)  [unwired: 1 in, 1 out]
  n4 = disable-structure shown="비활성화" {
    disable-tunnel: [w29 w31] -> w19
    disable-tunnel: w13 -> [w26 w31]
    frame Disabled {
      n5 = property on="Com_Status_Select" class="Enum (엄격한)"(error in=w26, "Val(Sgnl)"=T12."CHIP ID" ("값(신호)")) -> (error out=w28:errorcluster)  [unwired: 1 in, 1 out]
      n6 = property on="Read All" class="Bool (엄격한)"(error in=w28, "Val(Sgnl)"=FALSE ("값(신호)")) -> (error out=w29:errorcluster)  [unwired: 1 in, 1 out]
    }
    frame Enabled {
    }
  }
  n7 = control-ref of="Trig_Gen_Setting"() -> (w20:refnum<vi>)
  n8 = Build Array(w20) -> (w21:refnum<vi>[])
  n9 = call "(SubVI)Control Data_Save or Load Control Value.vi"("Val(Sgnl)"=TRUE, "Common? (f)"=TRUE, "Function"=(Ctrl)Control_Data_Save_or_Load_Control_Data_Function."Load", "error in (no error)"=w19, "Control Ref"=w21) -> ("error out"=w10:errorcluster)  [unwired: 6 in]
  n10 = global read "(Var)System Variables.vi" "Haptic IC"() -> (w11:refnum<class "Haptic IC.lvclass">)
  n11 = control-ref of="MEM_MODE"() -> (w7:refnum<vi>)
  n12 = control-ref of="Com_PWM_Freq"() -> (w9:refnum<vi>)
  n13 = control-ref of="Com_Bst_VD Clamp"() -> (w8:refnum<vi>)
  n14 = property class="Haptic IC.lvclass"(reference=w11, error in=w10, "Accessors:freq ref"=w9, "Accessors:voltage range ref"=w8, "Accessors:mode ref"=w7) -> (reference out=w6:refnum<class "Haptic IC.lvclass">, error out=w4:errorcluster)
  n15 = global write "(Var)System Variables.vi" "Haptic IC"(w6) -> ()
  n16 = property on="Com_PWM_Mode" class="Ring (엄격한)"(error in=w4, "DisabledEnum"=w2) -> (error out=w3:errorcluster)  [unwired: 1 in, 1 out]
  n17 = for {
    tunnel: cluster{string, u8}[] [{"Mem_Brake_Wave 0", 28}, {"Mem_Brake_Wave 1", 29}, {"AT_Track_Play", 53}, {"AT_Track_Idle", 54}, {"AT_Track_Wave 0", 55}, {"AT_Track_Wave 1", 56}, {"AT_Brake_Wave 0", 57}, {"AT_Brake_Wave 1", 58}] -> [w35] mode=indexing
    shift-right: [w32] -> w15
    shift-left: map{string, u8} {} ("맵 입력") -> [w36]
    n18 = Unbundle(w35) -> (w34:string, w33:u8)
    n19 = Insert Into Map(map in=w36, key=w34, value=w33) -> (map out=w32:map{string, u8})  [unwired: 2 out]
  }
  n20 = property on="Com_Bst_Wait" class="Ring (엄격한)"(error in=w3, "DisabledEnum"=w2) -> (error out=w1:errorcluster)  [unwired: 1 in, 1 out]
  n21 = while {
    tunnel: [w40] -> w23
    tunnel: w15 -> [w39]
    tunnel: w1 -> [_]
    stop <- w38 stop-if-true
    n22 = event shown="[8] \"Com_Bst_VD Clamp\": 값 변경" {
      selector: _ -> [_ _ _ _ _ _ _ _ _ _ _ _ _ _ _ _ _ _ _ _ _ _ _ _ _ _ _]
      dyn-events: _ -> [_ _ _ _ _ _ _ _ _ _ _ _ _ _ _ _ _ _ _ _ _ _ _ _ _ _ _]
      timeout: 100 -> [_ _ _ _ _ _ _ _ _ _ _ _ _ _ _ _ _ _ _ _ _ _ _ _ _ _ _]
      tunnel: [errorcluster {"status"=FALSE, "code"=0, "source"=""} ("에러 상수") _ _ _ _ _ _ _ _ _ _ _ _ _ _ _ _ _ _ _ _ _ _ _ _ _ _] -> w40
      tunnel: w39 -> [_ _ _ _ _ _ _ _ _ _ _ _ _ _ _ _ _ w584 _ _ _ _ _ _ _ _ _]
      event Timeout {
        n23 = event-data() -> ()  [unwired: 1 in, 3 out]
      }
      event "Com_Status_Select": Value Change {
        n24 = event-data() -> ()  [unwired: 1 in, 6 out]
        n25 = global read "(Var)System Variables.vi" "Main VI Log Ref"() -> (w45:refnum<vi>)
        n26 = global read "(Var)System Variables.vi" "IC I2C ID"() -> (w48:u8)
        n27 = Format Into String("Com_Status_Select") -> (resulting string=w47:string)  [unwired: 3 in, 1 out]
        n28 = call "(SubVI)I2C_Log_Append Header.vi"("Log Ref"=w45, "Header"=w47) -> ("error out"=w49:errorcluster)  [unwired: 9 in]
        n29 = case shown="\"Chip ID\", 기본" "Com_Status_Select" {
          tunnel: [w55 w67 w75 w94 w111 w143 w167 w177] -> w50
          tunnel: w49 -> [w52 w62 w72 w91 w135 w147 w152 w181]
          tunnel: w45 -> [w53 w63 w73 w92 w109 w138 w151 w172]
          tunnel: w48 -> [w54 w64 w74 w93 w110 w139 w150 w173]
          tunnel: [w51 w61 w71 w90 w136 w137 w149 w171] -> w44
          frame "Chip ID", Default {
            n30 = call-poly "(SubVI)I2C.vi"("Log Ref"=w53, "error in (no error)"=w52, "Address"=u8 0 ("Start Address"), "ID"=w54) -> ("error out"=w51:errorcluster, "Read Data"=w56:u8)  [unwired: 5 in, 1 out]
            n31 = call "(SubVI)Chip ID Converter.vi"("Chip ID"=w56) -> ("Chip Type"=w58:string)  [unwired: 10 in]
            n32 = Format Into String(format string=" / Info : 0x%02x" ("포맷 문자열"), initial string=w58, w56) -> (resulting string=w55:string)  [unwired: 1 in, 1 out]
          }
          frame "VBAT" {
            n33 = call-poly "(SubVI)I2C.vi"("Log Ref"=w63, "error in (no error)"=w62, "Address"=u8 8 ("Start Address"), "ID"=w64) -> ("error out"=w61:errorcluster, "Read Data"=w68:u8)  [unwired: 5 in, 1 out]
            n34 = To Unsigned Word Integer(number=w68) -> (unsigned 16bit integer=w60:u16)
            n35 = Multiply(x=w60, y=u16 40) -> (x*y=w66:u16)
            n36 = Format Into String(format string="VBAT : %dmV" ("포맷 문자열"), w66) -> (resulting string=w67:string)  [unwired: 2 in, 1 out]
          }
          frame "Status 0" {
            n37 = call-poly "(SubVI)I2C.vi"("Log Ref"=w73, "error in (no error)"=w72, "Address"=u8 1 ("Start Address"), "ID"=w74) -> ("error out"=w71:errorcluster, "Read Data"=w77:u8)  [unwired: 5 in, 1 out]
            n38 = case shown="1, 기본" w77 {
              selector: w77 -> [_ w87]
              tunnel: string[] ["SCP", "OCP", "TSD", "UVLO", "Process Done", "FIFO Empty", "FIFO Full", "TRIG In"] -> [_ w85]
              tunnel: ["Return 0" ("trimmed string") w80] -> w75
              frame 0 {
              }
              frame 1, Default {
                n39 = Number To Boolean Array(number=w87) -> (Boolean array=w86:bool[])
                n40 = for {
                  tunnel: w86 -> [w88] mode=indexing
                  tunnel: w85 -> [w89] mode=indexing
                  tunnel: [w89] -> w84 mode=indexing if=w88
                }
                n41 = Array To Spreadsheet String(delimiter (Tab)=" / " ("구분 문자 (탭)"), array=w84, 3:"%s" ("포맷 문자열")) -> (spreadsheet string=w81:string)
                n42 = call <vilib>:"Trim Whitespace.vi"("string"=w81) -> ("trimmed string"=w80:string)  [unwired: 1 in]
              }
            }
          }
          frame "Status 1" {
            n43 = call-poly "(SubVI)I2C.vi"("Log Ref"=w92, "error in (no error)"=w91, "Address"=u8 68 ("Start Address"), "ID"=w93) -> ("error out"=w90:errorcluster, "Read Data"=w96:u8)  [unwired: 5 in, 1 out]
            n44 = case shown="1, 기본" w96 {
              selector: w96 -> [_ w106]
              tunnel: string[] ["Active", "LRA Open", "TRIG1 R", "TRIG1 F", "TRIG2 R", "TRIG2 F", "TRIG3 R", "TRIG3 F"] -> [_ w104]
              tunnel: ["Return 0" ("trimmed string") w99] -> w94
              frame 0 {
              }
              frame 1, Default {
                n45 = Number To Boolean Array(number=w106) -> (Boolean array=w105:bool[])
                n46 = for {
                  tunnel: w105 -> [w107] mode=indexing
                  tunnel: w104 -> [w108] mode=indexing
                  tunnel: [w108] -> w103 mode=indexing if=w107
                }
                n47 = Array To Spreadsheet String(delimiter (Tab)=" / " ("구분 문자 (탭)"), array=w103, 3:"%s" ("포맷 문자열")) -> (spreadsheet string=w100:string)
                n48 = call <vilib>:"Trim Whitespace.vi"("string"=w100) -> ("trimmed string"=w99:string)  [unwired: 1 in]
              }
            }
          }
          frame "LRA F0 Value" {
            n49 = call-poly "(SubVI)I2C.vi"("Log Ref"=w109, "error in (no error)"=w135, "Size to Read"=u16 2, "Start Address"=u8 66, "ID"=w110) -> ("error out"=w136:errorcluster, "Read Data"=w131:u8[])  [unwired: 4 in, 1 out]
            n50 = Index Array(array=w131) -> (element #1=w130:u8, element #2=w122:u8)  [unwired: 2 in]
            n51 = Number To Boolean Array(number=w130) -> (Boolean array=w129:bool[])
            n52 = Index Array(array=w129, index #1=5 ("인덱스"), index #2=4 ("인덱스"), index #3=0 ("인덱스")) -> (element #1=w116:bool, element #2=w115:bool, element #3=w125:bool)
            n53 = Boolean To (0,1)(Boolean=w125) -> (0, 1=w124:i16)
            n54 = To Unsigned Byte Integer(number=w124) -> (unsigned 8bit integer=w123:u8)
            n55 = Join Numbers(hi=w123, lo=w122) -> ((hi.lo)=w121:u16)
            n56 = Format Into String(format string="Value : %d" ("포맷 문자열"), w121) -> (resulting string=w112:string)  [unwired: 2 in, 1 out]
            n57 = Select(t="Low Battery Voltage / ", s=w116, f="") -> (s? t:f=w114:string)
            n58 = Select(t="LRA F0 Freq. Error / ", s=w115, f="") -> (s? t:f=w113:string)
            n59 = Concatenate Strings(w114, w113, w112) -> (w111:string)
          }
          frame "FIFO Status" {
            n60 = call-poly "(SubVI)I2C.vi"("Log Ref"=w138, "error in (no error)"=w147, "Size to Read"=u16 2, "Start Address"=u8 77, "ID"=w139) -> ("error out"=w137:errorcluster, "Read Data"=w144:u8[])  [unwired: 4 in, 1 out]
            n61 = Type Cast(type=u16 0 ("타입"), x=w144) -> (*(type *) &x=w141:u16)
            n62 = Format Into String(format string="Value : %d" ("포맷 문자열"), w141) -> (resulting string=w143:string)  [unwired: 2 in, 1 out]
          }
          frame "RAM Checksum" {
            n63 = local read "Com_Mode"() -> (w160:T7)
            n64 = Unbundle(w160) -> ("MEM_MODE"=w159:bool, "DIAG_MODE"=w158:bool, "AUTO_BRAKE"=w157:bool, "AUTO_TRACK"=w156:bool)  [unwired: 2 out]
            n65 = Build Array(w159, w158, w157, w156, TRUE ("원소")) -> (w154:bool[])
            n66 = Boolean Array To Number ("불리언 배열을 숫자로")(Boolean array=w154) -> (number=w153:u8)
            n67 = call-poly "(SubVI)I2C.vi"("Log Ref"=w151, "error in (no error)"=w152, "Data to Write"=w153, "Address"=u8 11 ("Start Address"), "ID"=w150) -> ("error out"=w170:errorcluster)  [unwired: 5 in, 1 out]
            n68 = call-poly "(SubVI)I2C.vi"("Log Ref"=w151, "error in (no error)"=w170, "Size to Read"=u16 4, "Start Address"=u8 79, "ID"=w150) -> ("error out"=w149:errorcluster, "Read Data"=w164:u8[])  [unwired: 4 in, 1 out]
            n69 = Index Array(array=w164) -> (element #1=w163:u8, element #2=w162:u8, element #3=w161:u8, element #4=w148:u8)  [unwired: 4 in]
            n70 = Format Into String(format string="Checksum : %02x %02x %02x %02x" ("포맷 문자열"), w163, w162, w161, w148) -> (resulting string=w167:string)  [unwired: 2 in, 1 out]
          }
          frame "FIFO Level" {
            n71 = call-poly "(SubVI)I2C.vi"("Log Ref"=w172, "error in (no error)"=w181, "Size to Read"=u16 2, "Start Address"=u8 75, "ID"=w173) -> ("error out"=w171:errorcluster, "Read Data"=w178:u8[])  [unwired: 4 in, 1 out]
            n72 = Type Cast(type=u16 0 ("타입"), x=w178) -> (*(type *) &x=w175:u16)
            n73 = Format Into String(format string="FIFO Empty Value : %d Byte" ("포맷 문자열"), w175) -> (resulting string=w177:string)  [unwired: 2 in, 1 out]
          }
        }
        "Com_Status_Result" <- w50
        n74 = call "(SubVI)I2C_Log_Append LF.vi"("Log Ref"=w45, "error in (no error)"=w44) -> ()  [unwired: 9 in, 1 out]
      }
      event "Com_Status_Select": Operate Menu Activation; "Com_Status_Select": event #0x43 {
        # "현재 아이템과 동일한 아이템을 다시 선택해도\n값 변경 이벤트가 발생하도록\n열거형 클릭 시 임시로 값을 변경함\n\n값을 변경하지 않고 메뉴 해제 시 기존 값으로 다시 변경"
        n75 = event-data() -> ("CtlRef"=w187:refnum<vi>)  [unwired: 1 in, 3 out]
        n76 = property class="Enum (엄격한)"(reference=w187) -> (reference out=w184:refnum<vi>, error out=w185:errorcluster, "Value"=w186:T8)  [unwired: 1 in]
        n77 = feedback #1() -> (w182:T8)  [unwired: 1 in]
        n78 = case shown="\"\"" w186 {
          tunnel: w185 -> [w190 w193]
          tunnel: w184 -> [w191 w194]
          tunnel: [w189 w192] -> w183
          tunnel: w182 -> [_ w192]
          frame "Chip ID", Default {
            # "열거형 클릭 시 임시로 빈 문자열 아이템으로 변경,\n기존 값은 피드백 노드에 저장"
            n79 = property class="Enum (엄격한)"(reference=w191, error in=w190, "Value"=T8."" ("값")) -> ("Value"=w189:T8)  [unwired: 2 out]
          }
          frame "" {
            # "열거형 메뉴 해제 시 기존 값으로 다시 변경"
            n80 = property class="Enum (엄격한)"(reference=w194, error in=w193, "Value"=w192) -> ()  [unwired: 2 out]
          }
        }
        n81 = feedback-in #1(w183) -> ()
      }
      event "Read All": Value Change {
        w195 = FALSE ("값(신호)")
        # "Read All 버튼은 현재 사용하지 않음"
        # "값(신호) 프로퍼티 사용하기 위해\n스위치 모드로 사용"
        n82 = event-data() -> ()  [unwired: 1 in, 6 out]
        n83 = local write "Read All"(FALSE ("Read All")) -> ()
        n84 = property on="Com_Read" class="Bool (엄격한)"("Val(Sgnl)"=w195) -> (error out=w199:errorcluster)  [unwired: 2 in, 1 out]
        n85 = property on="Mem_Read" class="Bool (엄격한)"(error in=w199, "Val(Sgnl)"=w195) -> (error out=w197:errorcluster)  [unwired: 1 in, 1 out]
        n86 = property on="AT_Read" class="Bool (엄격한)"(error in=w197, "Val(Sgnl)"=w195) -> (error out=w196:errorcluster)  [unwired: 1 in, 1 out]
        n87 = property on="Trig_Read" class="Bool (엄격한)"(error in=w196, "Val(Sgnl)"=w195) -> ()  [unwired: 1 in, 2 out]
      }
      event "Com_Read", "Mem_Read", "AT_Read", "Trig_Read": Value Change {
        # "Read All 버튼으로 이벤트 발생했을 때\nI2C 에러가 발생할 경우 \n다음 이벤트를 발생시키지 않기 위함"
        # "값(신호) 프로퍼티 사용하기 위해\n스위치 모드로 사용"
        n88 = event-data() -> ("CtlRef"=w207:refnum<vi>)  [unwired: 1 in, 5 out]
        n89 = global read "(Var)System Variables.vi" "Main VI Log Ref"() -> (w201:refnum<vi>)
        n90 = property class="Bool (엄격한)"(reference=w207, "Value"=FALSE ("값")) -> ("Caption.Text"=w204:string)  [unwired: 1 in, 2 out]
        n91 = global read "(Var)System Variables.vi" "IC I2C ID"() -> (w203:u8)
        n92 = call "(SubVI)I2C_Log_Append Header.vi"("Log Ref"=w201, "Header"=w204) -> ("error out"=w205:errorcluster)  [unwired: 9 in]
        n93 = case shown="\"Trig Mode\"" w204 {
          tunnel: [w253 w309 w380 w402] -> w202
          tunnel: w205 -> [w215 w274 w333 w383]
          tunnel: w201 -> [w214 w273 w332 w381]
          tunnel: w203 -> [w213 w272 w331 w382]
          frame "Common", Default {
            n94 = call-poly "(SubVI)I2C.vi"("Log Ref"=w214, "error in (no error)"=w215, "Address to Read"=T13[] [{"Address"=11, "Delay(ms)"=0}, {"Address"=4, "Delay(ms)"=0}, {"Address"=7, "Delay(ms)"=0}, {"Address"=10, "Delay(ms)"=0}, {"Address"=6, "Delay(ms)"=0}], "ID"=w213) -> ("error out"=w253:errorcluster, "Read Data"=w251:u8[])  [unwired: 5 in, 1 out]
            n95 = Index Array(array=w251) -> (element #1=w250:u8, element #2=w248:u8, element #3=w247:u8, element #4=w242:u8, element #5=w239:u8)  [unwired: 6 in, 1 out]
            n96 = Number To Boolean Array(number=w250) -> (Boolean array=w209:bool[])
            n97 = Number To Boolean Array(number=w248) -> (Boolean array=w249:bool[])
            n98 = Number To Boolean Array(number=w247) -> (Boolean array=w246:bool[])
            n99 = Number To Boolean Array(number=w239) -> (Boolean array=w240:bool[])
            n100 = Array To Cluster(array=w209) -> (cluster=w227:T15)
            n101 = Index Array(array=w249) -> (element #1=w231:bool, element #2=w230:bool, element #3=w210:bool, element #4=w226:bool, element #5=w225:bool, element #6=w221:bool, element #7=w220:bool)  [unwired: 7 in]
            n102 = Split 1D Array(array=w246, index=4 ("인덱스")) -> (first subarray=w217:bool[], second subarray=w244:bool[])
            n103 = Split 1D Array(array=w240, index=4 ("인덱스")) -> (first subarray=w238:bool[], second subarray=w236:bool[])
            n104 = Index Array(array=w209) -> (element=w208:bool)  [unwired: 1 in]
            n105 = Boolean Array To Number ("불리언 배열을 숫자로")(Boolean array=w217) -> (number=w216:u8)
            n106 = Boolean Array To Number ("불리언 배열을 숫자로")(Boolean array=w244) -> (number=w243:u8)
            n107 = Boolean Array To Number ("불리언 배열을 숫자로")(Boolean array=w238) -> (number=w237:u8)
            n108 = Boolean Array To Number ("불리언 배열을 숫자로")(Boolean array=w236) -> (number=w235:u8)
            n109 = Build Array(w231, w230) -> (w229:bool[])
            n110 = Build Array(w226, w225) -> (w224:bool[])
            n111 = Build Array(w221, w220) -> (w219:bool[])
            n112 = Boolean Array To Number ("불리언 배열을 숫자로")(Boolean array=w229) -> (number=w228:u8)
            n113 = Boolean To (0,1)(Boolean=w210) -> (0, 1=w222:i16)
            n114 = Boolean Array To Number ("불리언 배열을 숫자로")(Boolean array=w224) -> (number=w223:u8)
            n115 = Boolean Array To Number ("불리언 배열을 숫자로")(Boolean array=w219) -> (number=w218:u8)
            n116 = In Range and Coerce(upper limit=u8 3 ("상위 리미트"), x=w235, lower limit=u8 0 ("하위 리미트")) -> (coerced(x)=w232:u8)  [unwired: 1 out]
            n117 = local write "Com_Mode"(w227) -> ()
            n118 = local write "Com_PWM_Freq"(w228) -> ()
            n119 = local write "Com_PWM_Mode"(w222) -> ()
            n120 = local write "Com_PWM_VHM"(w223) -> ()
            n121 = local write "Com_PWM_VD Time"(w218) -> ()
            n122 = local write "Com_Bst_Mode"(w216) -> ()
            n123 = local write "Com_Bst_Wait"(w243) -> ()
            n124 = local write "Com_Bst_VD Clamp"(w242) -> ()
            n125 = local write "Com_Bst_Offset"(w237) -> ()
            n126 = local write "Com_Bst_Limit"(w232) -> ()
            n127 = case shown="참" w208 {
              tunnel: [w254 T9."Enabled" ("비활성화")] -> w212
              tunnel: [w254 w256] -> w211
              tunnel: w210 -> [_ w255]
              frame False {
                w254 = T9."Disabled and Grayed Out" ("비활성화")
              }
              frame True {
                n128 = Select(t=T9."Enabled" ("비활성화"), s=w255, f=T9."Disabled and Grayed Out") -> (s? t:f=w256:T9)
              }
            }
            n129 = property on="Com_PWM_Mode" class="Ring (엄격한)"("DisabledEnum"=w212) -> ()  [unwired: 2 in, 2 out]
            n130 = property on="Com_Bst_Wait" class="Ring (엄격한)"("DisabledEnum"=w211) -> ()  [unwired: 2 in, 2 out]
          }
          frame "Memory Mode" {
            # "Wave Seq. 값에 따라 Mem No.와 Loop 링 아이템 변경"
            n131 = call-poly "(SubVI)I2C.vi"("Log Ref"=w273, "error in (no error)"=w274, "Size to Read"=u16 17, "Start Address"=u8 14, "ID"=w272) -> ("error out"=w309:errorcluster, "Read Data"=w297:u8[])  [unwired: 4 in, 1 out]
            n132 = Delete From Array(array=w297, index=0 ("인덱스")) -> (deleted portion=w260:u8, array with subset deleted=w269:u8[])  [unwired: 1 in]
            n133 = Split 1D Array(array=w269, index=12 ("인덱스")) -> (first subarray=w306:u8[], second subarray=w304:u8[])
            n134 = Index Array(array=w304) -> (element #1=w295:u8, element #2=w294:u8, element #3=w293:u8, element #4=w292:u8)  [unwired: 4 in]
            n135 = Split 1D Array(array=w306, index=8 ("길이")) -> (first subarray=w301:u8[], second subarray=w302:u8[])
            n136 = for {
              tunnel: w301 -> [w321] mode=indexing
              tunnel: [w315] -> w300 mode=indexing
              n137 = Number To Boolean Array(number=w321) -> (Boolean array=w320:bool[])
              n138 = Split 1D Array(array=w320, index=7 ("인덱스")) -> (first subarray=w318:bool[], second subarray=w317:bool[])
              n139 = Boolean Array To Number ("불리언 배열을 숫자로")(Boolean array=w318) -> (number=w316:u8)
              n140 = Boolean Array To Number ("불리언 배열을 숫자로")(Boolean array=w317) -> (number=w314:u8)
              n141 = Bundle(w314, w316) -> (w315:cluster{u8, u8})  [unwired: 1 in]
            }
            n142 = for {
              tunnel: w302 -> [w329] mode=indexing
              tunnel: [w322] -> w299 mode=concatenating
              n143 = Number To Boolean Array(number=w329) -> (Boolean array=w328:bool[])
              n144 = Split 1D Array(array=w328, index=4 ("인덱스")) -> (first subarray=w326:bool[], second subarray=w325:bool[])
              n145 = Boolean Array To Number ("불리언 배열을 숫자로")(Boolean array=w326) -> (number=w324:u8)
              n146 = Boolean Array To Number ("불리언 배열을 숫자로")(Boolean array=w325) -> (number=w323:u8)
              n147 = Build Array(w324, w323) -> (w322:u8[])
            }
            n148 = Number To Boolean Array(number=w292) -> (Boolean array=w291:bool[])
            n149 = Number To Boolean Array(number=w260) -> (Boolean array=w267:bool[])
            n150 = Index Array(array=w291) -> (element #1=w290:bool, element #2=w289:bool, element #3=w288:bool, element #4=w287:bool, element #5=w286:bool, element #6=w285:bool, element #7=w284:bool)  [unwired: 7 in]
            n151 = Index Array(array=w267) -> (element #1=w264:bool, element #2=w263:bool, element #3=w262:bool, element #4=w266:bool)  [unwired: 4 in]
            n152 = Build Array(w290, w289) -> (w283:bool[])
            n153 = Build Array(w288, w287, w286) -> (w282:bool[])
            n154 = Build Array(w285, w284) -> (w281:bool[])
            n155 = Build Array(w264, w263, w262) -> (w265:bool[])
            n156 = Boolean Array To Number ("불리언 배열을 숫자로")(Boolean array=w283) -> (number=w280:u8)
            n157 = Boolean Array To Number ("불리언 배열을 숫자로")(Boolean array=w282) -> (number=w279:u8)
            n158 = Boolean Array To Number ("불리언 배열을 숫자로")(Boolean array=w281) -> (number=w278:u8)
            n159 = Boolean Array To Number ("불리언 배열을 숫자로")(Boolean array=w265) -> (number=w261:u8)
            n160 = Array To Cluster(array=w300) -> (cluster=w277:T16)
            n161 = Array To Cluster(array=w299) -> (cluster=w298:T17)
            n162 = And(x=w295, y=u8 15) -> (x .and. y?=w303:u8)
            n163 = control-ref of="Mem Set_Wave Seq Loop"() -> (w270:refnum<vi>)
            n164 = control-ref of="Wave Seq. 0"() -> (w275:refnum<vi>)
            n165 = property on="Mem_Wave Seq" class="Clust (엄격한)"("Value"=w277) -> ("Controls[]"=w276:refnum<vi>[])  [unwired: 2 in, 2 out]
            n166 = local write "Mem Set_Wave Seq Loop"(w298) -> ()
            n167 = local write "Mem_Main Seq Loop"(w303) -> ()
            n168 = local write "Mem_Brake_Wave 0"(w294) -> ()
            n169 = local write "Mem_Brake_Wave 1"(w293) -> ()
            n170 = local write "Mem_Brake_Cycle 0"(w280) -> ()
            n171 = local write "Mem_Brake_Cycle 1"(w279) -> ()
            n172 = local write "Mem_Brake_VD"(w278) -> ()
            n173 = local write "Com_Bst_Mem Gain"(w261) -> ()
            n174 = local write "Com_Bst_Mute"(w266) -> ()
            n175 = for {
              tunnel: w276 -> [w312] mode=indexing
              tunnel: w275 -> [w311]
              tunnel: w270 -> [w310]
              n176 = To More Specific Class(target class=w311, reference=w312) -> (specific class reference=w313:refnum<vi>)  [unwired: 1 in, 1 out]
              n177 = call "(DW7912)Update Wave Seq Value Ring.vi"("Wave Seq Loop Ref In"=w310, "Wave Seq Ref In"=w313) -> ()  [unwired: 8 in, 2 out]
            }
          }
          frame "Auto Track Mode" {
            # "빈칸 :\n0x3C, 0x3D\nZXD_CTRL0,1"
            n178 = call-poly "(SubVI)I2C.vi"("Log Ref"=w332, "error in (no error)"=w333, "Size to Read"=u16 13, "Start Address"=u8 52, "ID"=w331) -> ("error out"=w380:errorcluster, "Read Data"=w379:u8[])  [unwired: 4 in, 1 out]
            n179 = Index Array(array=w379) -> (element #1=w367:u8, element #2=w363:u8, element #3=w362:u8, element #4=w361:u8, element #5=w360:u8, element #6=w359:u8, element #7=w358:u8, element #8=w351:u8, element #11=w341:u8, element #12=w338:u8, element #13=w335:u8)  [unwired: 13 in, 2 out]
            n180 = Number To Boolean Array(number=w367) -> (Boolean array=w374:bool[])
            n181 = Number To Boolean Array(number=w351) -> (Boolean array=w350:bool[])
            n182 = Number To Boolean Array(number=w341) -> (Boolean array=w342:bool[])
            n183 = And(x=w338, y=u8 1) -> (x .and. y?=w336:u8)
            n184 = Join Numbers(hi=w336, lo=w335) -> ((hi.lo)=w334:u16)
            n185 = Index Array(array=w374) -> (element #1=w373:bool, element #2=w372:bool, element #3=w375:bool, element #4=w371:bool, element #5=w370:bool, element #6=w376:bool, element #7=w377:bool, element #8=w366:bool)  [unwired: 8 in]
            n186 = Index Array(array=w350) -> (element #1=w352:bool, element #2=w353:bool, element #3=w349:bool, element #4=w354:bool, element #5=w355:bool, element #6=w348:bool, element #7=w347:bool)  [unwired: 7 in]
            n187 = Index Array(array=w342, index=1 ("인덱스")) -> (element=w339:bool)
            n188 = Build Array(w373, w372, w375) -> (w369:bool[])
            n189 = Build Array(w371, w370, w376, w377) -> (w368:bool[])
            n190 = Build Array(w352, w353) -> (w356:bool[])
            n191 = Build Array(w349, w354, w355) -> (w357:bool[])
            n192 = Build Array(w348, w347) -> (w346:bool[])
            n193 = Boolean Array To Number ("불리언 배열을 숫자로")(Boolean array=w369) -> (number=w365:u8)
            n194 = Boolean Array To Number ("불리언 배열을 숫자로")(Boolean array=w368) -> (number=w364:u8)
            n195 = Boolean Array To Number ("불리언 배열을 숫자로")(Boolean array=w356) -> (number=w345:u8)
            n196 = Boolean Array To Number ("불리언 배열을 숫자로")(Boolean array=w357) -> (number=w344:u8)
            n197 = Boolean Array To Number ("불리언 배열을 숫자로")(Boolean array=w346) -> (number=w343:u8)
            n198 = local write "AT_Track_Cycle 0"(w365) -> ()
            n199 = local write "AT_Track_Loop"(w364) -> ()
            n200 = local write "AT_Track_Pattern"(w366) -> ()
            n201 = local write "AT_Track_Play"(w363) -> ()
            n202 = local write "AT_Track_Idle"(w362) -> ()
            n203 = local write "AT_Track_Wave 0"(w361) -> ()
            n204 = local write "AT_Track_Wave 1"(w360) -> ()
            n205 = local write "AT_Brake_Wave 0"(w359) -> ()
            n206 = local write "AT_Brake_Wave 1"(w358) -> ()
            n207 = local write "AT_Brake_Cycle 0"(w345) -> ()
            n208 = local write "AT_Brake_Cycle 1"(w344) -> ()
            n209 = local write "AT_Brake_VD"(w343) -> ()
            n210 = local write "AT_LRA_F0"(w339) -> ()
            n211 = local write "AT_LRA_F0 In"(w334) -> ()
          }
          frame "Trig Mode" {
            n212 = call-poly "(SubVI)I2C.vi"("Log Ref"=w381, "error in (no error)"=w383, "Address"=u8 3, "ID"=w382) -> ("error out"=w404:errorcluster, "Read Data"=w401:u8)  [unwired: 5 in, 1 out]
            n213 = Number To Boolean Array(number=w401) -> (Boolean array=w400:bool[])
            n214 = call-poly "(SubVI)I2C.vi"("Log Ref"=w381, "error in (no error)"=w404, "Size to Read"=u16 21, "Start Address"=u8 31, "ID"=w382) -> ("error out"=w402:errorcluster, "Read Data"=w398:u8[])  [unwired: 4 in, 1 out]
            n215 = Index Array(array=w400) -> (element #1=w392:bool, element #2=w391:bool, element #3=w390:bool, element #4=w389:bool, element #5=w384:bool, element #6=w385:bool, element #7=w386:bool, element #8=w387:bool)  [unwired: 8 in]
            n216 = for {
              N: 3 -> [_]
              tunnel: w398 -> [w433]
              tunnel: [w407] -> w396 mode=indexing
              i -> [w432]
              n217 = Multiply(x=w432, y=7) -> (x*y=w431:i32)
              n218 = Index Array(array=w433, index #1=w431) -> (element #1=w428:u8, element #2=w427:u8, element #3=w426:u8, element #4=w425:u8, element #5=w424:u8, element #6=w423:u8, element #7=w422:u8)  [unwired: 6 in]
              n219 = Number To Boolean Array(number=w422) -> (Boolean array=w421:bool[])
              n220 = Index Array(array=w421) -> (element #1=w420:bool, element #2=w419:bool, element #3=w418:bool, element #4=w417:bool, element #5=w416:bool, element #6=w415:bool, element #7=w414:bool)  [unwired: 7 in]
              n221 = Build Array(w420, w419) -> (w413:bool[])
              n222 = Build Array(w418, w417, w416) -> (w412:bool[])
              n223 = Build Array(w415, w414) -> (w411:bool[])
              n224 = Boolean Array To Number ("불리언 배열을 숫자로")(Boolean array=w413) -> (number=w410:u8)
              n225 = Boolean Array To Number ("불리언 배열을 숫자로")(Boolean array=w412) -> (number=w409:u8)
              n226 = Boolean Array To Number ("불리언 배열을 숫자로")(Boolean array=w411) -> (number=w408:u8)
              n227 = Bundle(cluster=T6 {"TRIG R WAV"=0, "BRAKE0 R WAVE"=0, "BRAKE1 R WAVE"=0, "TRIG F WAV"=0, "BRAKE0 F WAVE"=0, "BRAKE1 F WAVE"=0, "BRAKE1 AT VD"=0, "BRAKE1 AT CYCLE"=0, "BRAKE0 AT CYCLE"=0} ("Trig_Wave_Trig 1"), "TRIG R WAV"=w428, "BRAKE0 R WAVE"=w427, "BRAKE1 R WAVE"=w426, "TRIG F WAV"=w425, "BRAKE0 F WAVE"=w424, "BRAKE1 F WAVE"=w423, "BRAKE1 AT VD"=w410, "BRAKE1 AT CYCLE"=w409, "BRAKE0 AT CYCLE"=w408) -> (w407:T6)
            }
            n228 = Build Array(w391, w390, w389) -> (w399:bool[])
            n229 = Boolean Array To Number(Boolean array=w399) -> (number=w388:u32)
            n230 = local write "Trig_Ctrl_Trig Priority"(w392) -> ()
            n231 = local write "Trig_Ctrl_Interval"(w388) -> ()
            n232 = local write "Trig_Ctrl_Trig1 Level"(w384) -> ()
            n233 = local write "Trig_Ctrl_Tirg1 Mode"(w385) -> ()
            n234 = local write "Trig_Ctrl_Trig2 Master"(w386) -> ()
            n235 = local write "Trig_Ctrl_Sound Mode"(w387) -> ()
            n236 = Index Array(array=w396) -> (element #1=w395:T6, element #2=w394:T6, element #3=w393:T6)  [unwired: 3 in]
            n237 = local write "Trig_Wave_Trig 1"(w395) -> ()
            n238 = local write "Trig_Wave_Trig 2"(w394) -> ()
            n239 = local write "Trig_Wave_Trig 3"(w393) -> ()
          }
        }
        n240 = call "(SubVI)I2C_Log_Append LF.vi"("Log Ref"=w201, "error in (no error)"=w202) -> ("error out"=w200:errorcluster)  [unwired: 9 in]
        n241 = case shown="에러 .." w200 {
          frame No Error {
          }
          frame Error {
            n242 = control-ref of="Com_Read"() -> (w437:refnum<vi>)
            n243 = control-ref of="Mem_Read"() -> (w436:refnum<vi>)
            n244 = control-ref of="AT_Read"() -> (w434:refnum<vi>)
            n245 = control-ref of="Trig_Read"() -> (w435:refnum<vi>)
            n246 = Build Array(w437, w436, w434, w435) -> (w438:refnum<vi>[])
            n247 = Flush Event Queue(2:w438) -> ()  [unwired: 5 in, 3 out]
          }
        }
      }
      event "Com_Mode": Value Change {
        w443 = FALSE ("값")
        # "두 불리언은 래치 성격임"
        n248 = event-data() -> ("NewVal"=w446:T7)  [unwired: 1 in, 5 out]
        n249 = disable-structure shown="활성화" {
          disable-tunnel: w446 -> [w460 w463]
          disable-tunnel: [w458 w463] -> w445
          disable-tunnel: [_ w463] -> w442
          frame Disabled {
            n250 = Unbundle By Name(w460) -> ("CHKSUM"=w462:bool, "MEM_MODE"=w461:bool)
            n251 = Or(x=w462, y=w461) -> (x .or. y?=w459:bool)
            n252 = Bundle By Name(cluster=w460, "MEM_MODE"=w459) -> (w458:T7)
          }
          frame Enabled {
          }
        }
        n253 = Unbundle By Name(w442) -> ("MEM_MODE"=w439:bool)
        n254 = global read "(Var)System Variables.vi" "Main VI Log Ref"() -> (w449:refnum<vi>)
        n255 = global read "(Var)System Variables.vi" "IC I2C ID"() -> (w450:u8)
        n256 = Cluster To Array(cluster=w445) -> (array=w447:bool[])
        n257 = case shown="참" w439 {
          tunnel: [w451 T9."Enabled" ("비활성화")] -> w441
          tunnel: [w451 w454] -> w440
          frame False {
            w451 = T9."Disabled and Grayed Out" ("비활성화")
          }
          frame True {
            n258 = local read "Com_PWM_Mode"() -> (w453:u8)
            n259 = Not Equal To 0?(x=w453) -> (x != 0?=w452:bool)
            n260 = Select(t=T9."Enabled" ("비활성화"), s=w452, f=T9."Disabled and Grayed Out") -> (s? t:f=w454:T9)
          }
        }
        n261 = Boolean Array To Number ("불리언 배열을 숫자로")(Boolean array=w447) -> (number=w444:u8)
        n262 = call-poly "(SubVI)I2C.vi"("Log Ref"=w449, "Data to Write"=w444, "Address"=u8 11, "ID"=w450) -> ()  [unwired: 6 in, 2 out]
        n263 = property on="FIFO_FLUSH" class="Bool (엄격한)"("Value"=w443) -> ()  [unwired: 2 in, 2 out]
        n264 = property on="CHKSUM" class="Bool (엄격한)"("Value"=w443) -> ()  [unwired: 2 in, 2 out]
        n265 = property on="Com_PWM_Mode" class="Ring (엄격한)"("DisabledEnum"=w441) -> ()  [unwired: 2 in, 2 out]
        n266 = property on="Com_Bst_Wait" class="Ring (엄격한)"("DisabledEnum"=w440) -> ()  [unwired: 2 in, 2 out]
      }
      event "Com_PWM_Freq", "Com_PWM_Mode", "Com_PWM_VHM", "Com_PWM_VD Time": Value Change {
        w471 = u8 0 items=["0", "1", "2", "3"] ("Com_PWM_VHM")
        # "Waveform Editor에서도 변경되도록 함"
        # "제거를 요청하여 숨김처리 함"
        n267 = event-data() -> ()  [unwired: 1 in, 6 out]
        n268 = Logical Shift(y=i16 2, x="Com_PWM_Mode") -> (x << y=w478:u8)
        n269 = Logical Shift(y=i16 3, x=w471) -> (x << y=w473:u8)
        n270 = Logical Shift(y=i16 5, x="Com_PWM_VD Time") -> (x << y=w472:u8)
        n271 = call "(SubVI)Waveform Editor_Update Sampling Rate Value.vi"("Action"=(Ctrl)Waveform_Editor_Update_Sampling_Rate_Value."Update", "Value"="Com_PWM_Freq") -> ()  [unwired: 9 in, 1 out]
        n272 = global read "(Var)System Variables.vi" "Main VI Log Ref"() -> (w481:refnum<vi>)
        n273 = Compound Arithmetic op=OR("Com_PWM_Freq", w478, w473, w472) -> (w477:u8)
        n274 = global read "(Var)System Variables.vi" "IC I2C ID"() -> (w482:u8)
        n275 = call-poly "(SubVI)I2C.vi"("Log Ref"=w481, "Data to Write"=w477, "Address"=u8 4, "ID"=w482) -> ()  [unwired: 6 in, 2 out]
        n276 = Not Equal To 0?(x="Com_PWM_Mode") -> (x != 0?=w468:bool)
        n277 = Select(t=T9."Enabled" ("비활성화"), s=w468, f=T9."Disabled and Grayed Out") -> (s? t:f=w464:T9)
        n278 = property on="Com_Bst_Wait" class="Ring (엄격한)"("DisabledEnum"=w464) -> ()  [unwired: 2 in, 2 out]
      }
      event "Com_Bst_Mode", "Com_Bst_Wait": Value Change {
        n279 = event-data() -> ()  [unwired: 1 in, 6 out]
        n280 = Logical Shift(y=i16 4, x="Com_Bst_Wait") -> (x << y=w486:u8)
        n281 = global read "(Var)System Variables.vi" "Main VI Log Ref"() -> (w489:refnum<vi>)
        n282 = Or(x="Com_Bst_Mode", y=w486) -> (x .or. y?=w485:u8)
        n283 = global read "(Var)System Variables.vi" "IC I2C ID"() -> (w490:u8)
        n284 = call-poly "(SubVI)I2C.vi"("Log Ref"=w489, "Data to Write"=w485, "Address"=u8 7, "ID"=w490) -> ()  [unwired: 6 in, 2 out]
      }
      event "Com_Bst_VD Clamp": Value Change {
        n285 = event-data() -> ()  [unwired: 1 in, 6 out]
        n286 = global read "(Var)System Variables.vi" "Main VI Log Ref"() -> (w493:refnum<vi>)
        n287 = global read "(Var)System Variables.vi" "IC I2C ID"() -> (w494:u8)
        n288 = call-poly "(SubVI)I2C.vi"("Log Ref"=w493, "Data to Write"="Com_Bst_VD Clamp", "Address"=u8 10, "ID"=w494) -> ()  [unwired: 6 in, 2 out]
      }
      event "Com_Bst_Limit", "Com_Bst_Offset": Value Change {
        n289 = event-data() -> ()  [unwired: 1 in, 6 out]
        n290 = disable-structure shown="활성화" {
          disable-tunnel: [w503 w506] -> w497
          disable-tunnel: "Com_Bst_Offset" -> [w502 w506]
          disable-tunnel: "Com_Bst_Limit" -> [w501 _]
          frame Enabled {
            n291 = Logical Shift(y=i16 4, x=w501) -> (x << y=w504:u8)
            n292 = Or(x=w502, y=w504) -> (x .or. y?=w503:u8)
          }
          frame Disabled {
          }
        }
        n293 = global read "(Var)System Variables.vi" "Main VI Log Ref"() -> (w499:refnum<vi>)
        n294 = global read "(Var)System Variables.vi" "IC I2C ID"() -> (w500:u8)
        n295 = call-poly "(SubVI)I2C.vi"("Log Ref"=w499, "Data to Write"=w497, "Address"=u8 6, "ID"=w500) -> ()  [unwired: 6 in, 2 out]
      }
      event "Com_Bst_Mem Gain", "Com_Bst_Mute": Value Change {
        n296 = event-data() -> ()  [unwired: 1 in, 6 out]
        n297 = Boolean To (0,1)(Boolean="Com_Bst_Mute") -> (0, 1=w511:i16)
        n298 = To Unsigned Byte Integer(number=w511) -> (unsigned 8bit integer=w510:u8)
        n299 = Logical Shift(y=i16 3, x=w510) -> (x << y=w513:u8)
        n300 = global read "(Var)System Variables.vi" "Main VI Log Ref"() -> (w515:refnum<vi>)
        n301 = Or(x="Com_Bst_Mem Gain", y=w513) -> (x .or. y?=w507:u8)
        n302 = global read "(Var)System Variables.vi" "IC I2C ID"() -> (w516:u8)
        n303 = call-poly "(SubVI)I2C.vi"("Log Ref"=w515, "Data to Write"=w507, "Address"=u8 14, "ID"=w516) -> ()  [unwired: 6 in, 2 out]
      }
      event Value Change {
        # "Wave Seq. 0 주소\n원소의 인덱스에 따라 주소를 증가"
        n304 = event-data() -> ("CtlRef"=w529:refnum<vi>)  [unwired: 1 in, 5 out]
        n305 = property class="Clust (엄격한)"(reference=w529) -> (reference out=w518:refnum<vi>, "Value"=w517:T3)  [unwired: 1 in, 1 out]
        n306 = control-ref of="Mem Set_Wave Seq Loop"() -> (w519:refnum<vi>)
        n307 = Unbundle(w517) -> ("Mode"=w521:u8, "Seq/Delay"=w526:u8)
        n308 = call "(DW7912)Update Wave Seq Value Ring.vi"("Wave Seq Loop Ref In"=w519, "Wave Seq Ref In"=w518) -> ("index"=w520:u8)  [unwired: 8 in, 1 out]
        n309 = Logical Shift(y=i16 7, x=w521) -> (x << y=w527:u8)
        n310 = Or(x=w527, y=w526) -> (x .or. y?=w525:u8)
        n311 = Add(x=w520, y=u8 15) -> (x+y=w524:u8)
        n312 = global read "(Var)System Variables.vi" "Main VI Log Ref"() -> (w522:refnum<vi>)
        n313 = global read "(Var)System Variables.vi" "IC I2C ID"() -> (w523:u8)
        n314 = call-poly "(SubVI)I2C.vi"("Log Ref"=w522, "Data to Write"=w525, "Address"=w524, "ID"=w523) -> ()  [unwired: 6 in, 2 out]
      }
      event Value Change {
        w536 = refnum<vi> refnum  # 클러스터
        # "FAE3팀에서 Wave Seq.의 Mode 변경 시 \nMem.No의 값을 0으로 변경하도록 요청"
        n315 = event-data() -> ("CtlRef"=w531:refnum<vi>)  [unwired: 1 in, 5 out]
        n316 = property class="Ring (엄격한)"(reference=w531) -> ("Owner"=w538:refnum<vi>)  [unwired: 1 in, 2 out]
        n317 = To More Specific Class(target class=w536, reference=w538) -> (specific class reference=w537:refnum<vi>)  [unwired: 1 in, 1 out]
        n318 = property class="Clust"(reference=w537) -> ("Controls[]"=w535:refnum<vi>[])  [unwired: 1 in, 2 out]
        n319 = Index Array(array=w535, index=1 ("인덱스")) -> (element=w533:refnum<vi>)
        n320 = property class="Ctl"(reference=w533, "Value"=u8 0) -> ()  [unwired: 1 in, 2 out]
      }
      event "Mem Set_Wave Seq Loop.Loop 0", "Mem Set_Wave Seq Loop.Loop 1", "Mem Set_Wave Seq Loop.Loop 2", "Mem Set_Wave Seq Loop.Loop 3", "Mem Set_Wave Seq Loop.Loop 4", "Mem Set_Wave Seq Loop.Loop 5", "Mem Set_Wave Seq Loop.Loop 6", "Mem Set_Wave Seq Loop.Loop 7": Value Change {
        # "Wave Seq Loop의 경우 2개가 1바이트"
        n321 = event-data() -> ("CtlRef"=w550:refnum<vi>)  [unwired: 1 in, 5 out]
        n322 = property on="Mem Set_Wave Seq Loop" class="Clust (엄격한)"() -> ("Controls[]"=w555:refnum<vi>[])  [unwired: 2 in, 2 out]
        n323 = call "Search Unsorted 1D Array.vim"("element"=w550, "unsorted 1D array"=w555) -> ("index of element"=w554:i32)  [unwired: 9 in]
        n324 = Cluster To Array(cluster="Mem Set_Wave Seq Loop") -> (array=w547:u8[])
        n325 = To Unsigned Byte Integer(number=w554) -> (unsigned 8bit integer=w556:u8)
        n326 = Quotient & Remainder(x=w556, y=u8 2) -> (floor(x/y)=w546:u8)  [unwired: 1 out]
        n327 = Multiply(x=w546, y=u8 2) -> (x*y=w540:u8)
        n328 = Add(x=w546, y=u8 23) -> (x+y=w553:u8)
        n329 = Index Array(array=w547, index #1=w540) -> (element #1=w543:u8, element #2=w545:u8)  [unwired: 1 in]
        n330 = global read "(Var)System Variables.vi" "Main VI Log Ref"() -> (w551:refnum<vi>)
        n331 = global read "(Var)System Variables.vi" "IC I2C ID"() -> (w552:u8)
        n332 = Logical Shift(y=i16 4, x=w545) -> (x << y=w542:u8)
        n333 = Or(x=w543, y=w542) -> (x .or. y?=w541:u8)
        n334 = call-poly "(SubVI)I2C.vi"("Log Ref"=w551, "Data to Write"=w541, "Address"=w553, "ID"=w552) -> ()  [unwired: 6 in, 2 out]
      }
      event "Mem_Main Seq Loop": Value Change {
        n335 = event-data() -> ()  [unwired: 1 in, 6 out]
        n336 = global read "(Var)System Variables.vi" "Main VI Log Ref"() -> (w560:refnum<vi>)
        n337 = global read "(Var)System Variables.vi" "IC I2C ID"() -> (w561:u8)
        n338 = call-poly "(SubVI)I2C.vi"("Log Ref"=w560, "Data to Write"="Mem_Main Seq Loop", "Address"=u8 27, "ID"=w561) -> ()  [unwired: 6 in, 2 out]
      }
      event "Mem_Start", "Mem_Stop", "AT_Start", "AT_Stop": Value Change {
        # "Stop 이벤트 시 0\nStart 이벤트 시 1"
        n339 = event-data() -> ()  [unwired: 1 in, 6 out]
        n340 = Or(x="Mem_Start", y="AT_Start") -> (x .or. y?=w563:bool)
        n341 = Boolean To (0,1)(Boolean=w563) -> (0, 1=w566:i16)
        n342 = To Unsigned Byte Integer(number=w566) -> (unsigned 8bit integer=w565:u8)
        n343 = global read "(Var)System Variables.vi" "Main VI Log Ref"() -> (w568:refnum<vi>)
        n344 = global read "(Var)System Variables.vi" "IC I2C ID"() -> (w569:u8)
        n345 = call-poly "(SubVI)I2C.vi"("Log Ref"=w568, "Data to Write"=w565, "Address"=u8 12, "ID"=w569) -> ()  [unwired: 6 in, 2 out]
      }
      event "Mem_Brake_Cycle 0", "Mem_Brake_Cycle 1", "Mem_Brake_VD": Value Change {
        n346 = event-data() -> ()  [unwired: 1 in, 6 out]
        n347 = Logical Shift(y=i16 2, x="Mem_Brake_Cycle 1") -> (x << y=w574:u8)
        n348 = Logical Shift(y=i16 5, x="Mem_Brake_VD") -> (x << y=w573:u8)
        n349 = global read "(Var)System Variables.vi" "Main VI Log Ref"() -> (w579:refnum<vi>)
        n350 = global read "(Var)System Variables.vi" "IC I2C ID"() -> (w580:u8)
        n351 = Compound Arithmetic op=OR("Mem_Brake_Cycle 0", w574, w573) -> (w575:u8)
        n352 = call-poly "(SubVI)I2C.vi"("Log Ref"=w579, "Data to Write"=w575, "Address"=u8 30, "ID"=w580) -> ()  [unwired: 6 in, 2 out]
      }
      event "Mem_Brake_Wave 0", "Mem_Brake_Wave 1", "AT_Track_Play", "AT_Track_Idle", "AT_Track_Wave 0", "AT_Track_Wave 1", "AT_Brake_Wave 0", "AT_Brake_Wave 1": Value Change {
        # "컨트롤 1개가 레지스터 1개의 값인 경우\n코드를 간단하게 하기위해 맵을 사용하였음"
        n353 = event-data() -> ("CtlRef"=w585:refnum<vi>, "NewVal"=w582:u8)  [unwired: 1 in, 4 out]
        n354 = property class="Ring (엄격한)"(reference=w585) -> ("Label.Text"=w583:string)  [unwired: 1 in, 2 out]
        n355 = Look In Map(map=w584, key=w583) -> (value=w581:u8)  [unwired: 1 in, 1 out]
        n356 = global read "(Var)System Variables.vi" "Main VI Log Ref"() -> (w586:refnum<vi>)
        n357 = global read "(Var)System Variables.vi" "IC I2C ID"() -> (w587:u8)
        n358 = call-poly "(SubVI)I2C.vi"("Log Ref"=w586, "Data to Write"=w582, "Address"=w581, "ID"=w587) -> ()  [unwired: 6 in, 2 out]
      }
      event "AT_Track_Pattern", "AT_Track_Loop", "AT_Track_Cycle 0": Value Change {
        n359 = event-data() -> ()  [unwired: 1 in, 6 out]
        n360 = Boolean To (0,1)(Boolean="AT_Track_Pattern") -> (0, 1=w597:i16)
        n361 = To Unsigned Byte Integer(number=w597) -> (unsigned 8bit integer=w591:u8)
        n362 = Logical Shift(y=i16 3, x="AT_Track_Loop") -> (x << y=w589:u8)
        n363 = Logical Shift(y=i16 7, x=w591) -> (x << y=w588:u8)
        n364 = global read "(Var)System Variables.vi" "Main VI Log Ref"() -> (w599:refnum<vi>)
        n365 = global read "(Var)System Variables.vi" "IC I2C ID"() -> (w600:u8)
        n366 = Compound Arithmetic op=OR("AT_Track_Cycle 0", w589, w588) -> (w590:u8)
        n367 = call-poly "(SubVI)I2C.vi"("Log Ref"=w599, "Data to Write"=w590, "Address"=u8 52, "ID"=w600) -> ()  [unwired: 6 in, 2 out]
      }
      event "AT_Brake_Cycle 0", "AT_Brake_Cycle 1", "AT_Brake_VD": Value Change {
        n368 = event-data() -> ()  [unwired: 1 in, 6 out]
        n369 = Logical Shift(y=i16 2, x="AT_Brake_Cycle 1") -> (x << y=w605:u8)
        n370 = Logical Shift(y=i16 5, x="AT_Brake_VD") -> (x << y=w604:u8)
        n371 = global read "(Var)System Variables.vi" "Main VI Log Ref"() -> (w610:refnum<vi>)
        n372 = global read "(Var)System Variables.vi" "IC I2C ID"() -> (w611:u8)
        n373 = Compound Arithmetic op=OR("AT_Brake_Cycle 0", w605, w604) -> (w606:u8)
        n374 = call-poly "(SubVI)I2C.vi"("Log Ref"=w610, "Data to Write"=w606, "Address"=u8 59, "ID"=w611) -> ()  [unwired: 6 in, 2 out]
      }
      event "AT_LRA_F0": Value Change {
        n375 = event-data() -> ()  [unwired: 1 in, 6 out]
        n376 = Boolean To (0,1)(Boolean="AT_LRA_F0") -> (0, 1=w616:i16)
        n377 = To Unsigned Byte Integer(number=w616) -> (unsigned 8bit integer=w615:u8)
        n378 = Logical Shift(y=i16 1, x=w615) -> (x << y=w612:u8)
        n379 = global read "(Var)System Variables.vi" "Main VI Log Ref"() -> (w618:refnum<vi>)
        n380 = global read "(Var)System Variables.vi" "IC I2C ID"() -> (w619:u8)
        n381 = call-poly "(SubVI)I2C.vi"("Log Ref"=w618, "Data to Write"=w612, "Address"=u8 62, "ID"=w619) -> ()  [unwired: 6 in, 2 out]
      }
      event "AT_LRA_F0 In": Value Change {
        w621 = u8[] []  # U8
        n382 = event-data() -> ()  [unwired: 1 in, 6 out]
        n383 = Type Cast(type=w621, x="AT_LRA_F0 In") -> (*(type *) &x=w620:u8[])
        n384 = global read "(Var)System Variables.vi" "Main VI Log Ref"() -> (w624:refnum<vi>)
        n385 = global read "(Var)System Variables.vi" "IC I2C ID"() -> (w625:u8)
        n386 = call-poly "(SubVI)I2C.vi"("Log Ref"=w624, "Data to Write"=w620, "Start Address"=u8 63 ("Address"), "ID"=w625) -> ()  [unwired: 6 in, 2 out]
      }
      event "Trig_Ctrl_Trig Priority", "Trig_Ctrl_Interval", "Trig_Ctrl_Trig1 Level", "Trig_Ctrl_Tirg1 Mode", "Trig_Ctrl_Trig2 Master", "Trig_Ctrl_Sound Mode": Value Change {
        # "제거를 요청하여 숨김처리 함"
        n387 = event-data() -> ()  [unwired: 1 in, 6 out]
        n388 = Number To Boolean Array(number="Trig_Ctrl_Interval") -> (Boolean array=w636:bool[])
        n389 = Index Array(array=w636) -> (element #1=w634:bool, element #2=w633:bool, element #3=w632:bool)  [unwired: 3 in]
        n390 = global read "(Var)System Variables.vi" "Main VI Log Ref"() -> (w639:refnum<vi>)
        n391 = Build Array("Trig_Ctrl_Trig Priority", w634, w633, w632, "Trig_Ctrl_Trig1 Level", "Trig_Ctrl_Tirg1 Mode", "Trig_Ctrl_Trig2 Master", FALSE) -> (w628:bool[])
        n392 = global read "(Var)System Variables.vi" "IC I2C ID"() -> (w640:u8)
        n393 = Boolean Array To Number ("불리언 배열을 숫자로")(Boolean array=w628) -> (number=w627:u8)
        n394 = call-poly "(SubVI)I2C.vi"("Log Ref"=w639, "Data to Write"=w627, "Address"=u8 3, "ID"=w640) -> ()  [unwired: 6 in, 2 out]
      }
      event Value Change {
        # "이 이벤트 케이스는 클러스터 원소 중 아래  컨트롤만 해당\n\nTRIG R Wave\nTRIG F Wave\nBrake0 R Wave\nBrake1 F Wave\nBrake1 R Wave\nBrake1 F Wave"
        # "TRIG1 레지스터 시작 주소"
        # "각 클러스터마다 레지스터가 7개임"
        # "소유자 클러스터의 라벨"
        # "탭으로 되어있음"
        n395 = event-data() -> ("CtlRef"=w657:refnum<vi>, "NewVal"=w643:u8)  [unwired: 1 in, 4 out]
        n396 = property class="Ring (엄격한)"(reference=w657) -> (reference out=w653:refnum<vi>, "Owner"=w656:refnum<vi>)  [unwired: 1 in, 1 out]
        n397 = control-ref of="Trig_Wave_Trig 1"() -> (w642:refnum<vi>)
        n398 = To More Specific Class(target class=w642, reference=w656) -> (specific class reference=w655:refnum<vi>)  [unwired: 1 in, 1 out]
        n399 = property class="Clust (엄격한)"(reference=w655) -> ("Label.Text"=w652:string, "Controls[]"=w654:refnum<vi>[])  [unwired: 1 in, 2 out]
        n400 = call "Search Unsorted 1D Array.vim"("element"=w653, "unsorted 1D array"=w654) -> ("index of element"=w646:i32)  [unwired: 9 in]
        n401 = Scan From String(format string="Trig_Wave_Trig %d" ("포맷 문자열"), input string=w652) -> (output 1=w650:i32)  [unwired: 3 in, 3 out]
        n402 = Decrement(x=w650) -> (x-1=w641:i32)
        n403 = Multiply(x=7, y=w641) -> (x*y=w648:i32)
        n404 = Compound Arithmetic op=ADD(w648, 31 ("값"), w646) -> (w645:i32)
        n405 = To Unsigned Byte Integer(number=w645) -> (unsigned 8bit integer=w644:u8)
        n406 = global read "(Var)System Variables.vi" "Main VI Log Ref"() -> (w658:refnum<vi>)
        n407 = global read "(Var)System Variables.vi" "IC I2C ID"() -> (w659:u8)
        n408 = call-poly "(SubVI)I2C.vi"("Log Ref"=w658, "Data to Write"=w643, "Address"=w644, "ID"=w659) -> ()  [unwired: 6 in, 2 out]
      }
      event Value Change {
        # "각 클러스터마다 레지스터가 7개임"
        # "소유자 클러스터의 라벨"
        # "이 이벤트 케이스는 클러스터 원소 중 아래  컨트롤만 해당\n\nBrake0 T Cycle\nBrake1 T Cycle\nBrake1 T VD"
        n409 = event-data() -> ("CtlRef"=w681:refnum<vi>)  [unwired: 1 in, 5 out]
        n410 = property class="Ring (엄격한)"(reference=w681) -> ("Owner"=w680:refnum<vi>)  [unwired: 1 in, 2 out]
        n411 = control-ref of="Trig_Wave_Trig 1"() -> (w669:refnum<vi>)
        n412 = To More Specific Class(target class=w669, reference=w680) -> (specific class reference=w679:refnum<vi>)  [unwired: 1 in, 1 out]
        n413 = property class="Clust (엄격한)"(reference=w679) -> ("Label.Text"=w678:string, "Value"=w670:T6)  [unwired: 1 in, 2 out]
        n414 = Unbundle By Name(w670) -> ("BRAKE1 AT VD"=w664:u8, "BRAKE1 AT CYCLE"=w668:u8, "BRAKE0 AT CYCLE"=w665:u8)
        n415 = Scan From String(format string="Trig_Wave_Trig %d" ("포맷 문자열"), input string=w678) -> (output 1=w676:i32)  [unwired: 3 in, 3 out]
        n416 = Decrement(x=w676) -> (x-1=w660:i32)
        n417 = Multiply(x=7, y=w660) -> (x*y=w674:i32)
        n418 = Logical Shift(y=i16 2, x=w668) -> (x << y=w663:u8)
        n419 = Logical Shift(y=i16 5, x=w665) -> (x << y=w662:u8)
        n420 = Compound Arithmetic op=ADD(w674, 37 ("값")) -> (w672:i32)
        n421 = To Unsigned Byte Integer(number=w672) -> (unsigned 8bit integer=w671:u8)
        n422 = Compound Arithmetic op=OR(w664, w663, w662) -> (w661:u8)
        n423 = global read "(Var)System Variables.vi" "Main VI Log Ref"() -> (w682:refnum<vi>)
        n424 = global read "(Var)System Variables.vi" "IC I2C ID"() -> (w683:u8)
        n425 = call-poly "(SubVI)I2C.vi"("Log Ref"=w682, "Data to Write"=w661, "Address"=w671, "ID"=w683) -> ()  [unwired: 6 in, 2 out]
      }
      event Value Change {
        # "Trigger 설정에 따른 그림 생성"
        # "비활성화, 시간 설정 범위 관련 처리"
        n426 = event-data() -> ("CtlRef"=w688:refnum<vi>)  [unwired: 1 in, 5 out]
        n427 = call "(SubVI)Update Trigger Control Cluster.vi"("Trig Ctrl Ref"=w688) -> ("Disable"=w687:T9)  [unwired: 9 in, 1 out]
        n428 = property on="Trig_Gen_Set" class="Bool"("DisabledEnum"=w687) -> ()  [unwired: 2 in, 2 out]
        n429 = call "(SubVI)GPIO Trigger Picture.vi"("num of ch (4)"=3, "Trig Ctrl"="Trig_Gen_Setting") -> ("picture"=→"Trig_Gen_Pict":picture)  [unwired: 9 in]
      }
      event "Trig_Gen_Set": Value Change {
        # "트리거 발생"
        n430 = event-data() -> ()  [unwired: 1 in, 6 out]
        n431 = local read "Trig_Gen_Setting"() -> (w689:T5)
        n432 = call "(SubVI)System Command_Trig GPIO Control.vi"("Trig_Ctrl"=w689) -> ()  [unwired: 10 in, 1 out]
      }
    }
    n433 = global read "(Var)System Variables.vi" "Quit System"() -> (w41:bool)
    n434 = Or(x="Stop", y=w41) -> (x .or. y?=w38:bool)
  }
  n435 = flat-sequence {
    tunnel: w23 -> [_]
    frame #0 {
      # "Trigger 설정 값 저장"
      n436 = control-ref of="Trig_Gen_Setting"() -> (w693:refnum<vi>)
      n437 = Build Array(w693) -> (w692:refnum<vi>[])
      n438 = call "(SubVI)Control Data_Save or Load Control Value.vi"("Common? (f)"=TRUE, "Function"=(Ctrl)Control_Data_Save_or_Load_Control_Data_Function."Save", "Control Ref"=w692) -> ()  [unwired: 8 in, 1 out]
    }
  }
